vi "newMicroTime.vi"() -> ()   [LabVIEW 2013]
uses:
  Camera/vi/GlobalSetGetConfigureCamera.vi
  Variables/GetPicture.vi
  Variables/GlobalLaserInterface.vi
  Variables/patternImg.vi
panel:
  in  "Tab Control":T1(tab)
  out "Histogram":i32[][](graph)
  out "Trace":i32[][](graph)=[[2, 0, 0, 1, 1, 1, 0, 0, 0, 1, 0, 1, 0, 1, 2, 2, 0, 3, 0, 2, 2, 1, 3, 1, 0, 1, 1, 1, 0, 1, 3, 1, 0, 2, 0, 1, 0, 1, 1, 0, 1, 1, 3, 1, 0, 2, 0, 1, 1, 0, 0, 2, 0, 0, 1, 1, 1, 0, 0, 1, 0, 1, 0, 0, 0, 1, 2, 1, 1, 2, 0, 2, 4, 3, 1, 1, 0, 0, 1, 1, 2, 0, 1, 1, 0, 0, 0, 1, 1, 1, 1, 3, 0, 0, 1, 0, 0, 0, 2, 1, 1, 1, 2, 1, 0, 1, 1, 0, 0, 2, 1, 1, 0, 0, 1, 1, 1, 1, 0, 2, 2, 0, 1, 2, 1, 0, 3, 0, 2, 1, 3, 0, 1, 1, 0, 0, 3, 0, 0, 0, 0, 0, 0, 0, 0, 0, 0, 0, 0, 0, 0, 0, 0, 0, 0, 0, 0, 0, 0, 0, 0, 0, 0, 0, 0, 0, 0, 0, 0, 0, 0, 0, 0, 0, 0, 0, 0, 0, 0, 0, 0, 0, 0, 0, 0, 0, 0, 0, 0, 0, 0, 0, 0, 0, 0, 0, 0, 0, 0, 0], [1, 2, 2, 0, 0, 0, 1, 2, 1, 2, 1, 1, 1, 0, 0, 0, 3, 1, 0, 1, 0, 2, 0, 2, 1, 1, 0, 0, 1, 0, 1, 2, 1, 0, 0, 0, 0, 0, 1, 0, 1, 0, 2, 0, 1, 0, 0, 0, 0, 1, 1, 3, 0, 0, 0, 2, 0, 0, 2, 0, 1, 1, 0, 0, 2, 0, 2, 1, 0, 1, 1, 0, 1, 1, 0, 0, 0, 1, 0, 0, 1, 0, 0, 0, 0, 1, 0, 1, 1, 1, 1, 0, 0, 0, 1, 1, 1, 0, 1, 0, 0, 0, 1, 1, 1, 0, 0, 1, 1, 3, 1, 0, 0, 0, 0, 0, 0, 0, 1, 2, 1, 0, 0, 0, 2, 3, 3, 2, 0, 1, 1, 1, 0, 0, 4, 0, 1, 2, 0, 0, 0, 2, 0, 0, 0, 0, 0, 0, 0, 0, 0, 0, 0, 0, 0, 0, 0, 0, 0, 0, 0, 0, 0, 0, 0, 0, 0, 0, 0, 0, 0, 0, 0, 0, 0, 0, 0, 0, 0, 0, 0, 0, 0, 0, 0, 0, 0, 0, 0, 0, 0, 0, 0, 0, 0, 0, 0, 0, 0, 0], [2, 2, 0, 1, 2, 0, 1, 0, 2, 3, 1, 0, 1, 0, 1, 0, 0, 0, 0, 2, 1, 0, 0, 2, 2, 0, 0, 0, 3, 0, 0, 2, 2, 2, 0, 3, 0, 3, 1, 3, 1, 3, 1, 0, 3, 1, 3, 3, 1, 1, 1, 1, 2, 0, 1, 0, 1, 1, 1, 3, 0, 2, 3, 1, 1, 1, 0, 1, 0, 1, 2, 3, 1, 2, 1, 3, 0, 2, 0, 2, 0, 1, 0, 2, 2, 1, 1, 3, 1, 2, 1, 1, 1, 3, 0, 0, 0, 0, 1, 1, 1, 0, 1, 0, 2, 1, 1, 0, 1, 0, 1, 2, 2, 2, 2, 0, 1, 0, 0, 0, 1, 1, 2, 0, 0, 1, 5, 2, 2, 0, 2, 0, 2, 2, 2, 0, 1, 0, 6, 0, 0, 0, 0, 0, 0, 0, 0, 0, 0, 0, 0, 0, 0, 0, 0, 0, 0, 0, 0, 0, 0, 0, 0, 0, 0, 0, 0, 0, 0, 0, 0, 0, 0, 0, 0, 0, 0, 0, 0, 0, 0, 0, 0, 0, 0, 0, 0, 0, 0, 0, 0, 0, 0, 0, 0, 0, 0, 0, 0, 0], [0, 0, 1, 0, 1, 1, 0, 0, 0, 1, 1, 0, 1, 0, 0, 0, 0, 0, 2, 0, 0, 0, 0, 2, 0, 0, 0, 1, 1, 2, 1, 1, 1, 2, 1, 0, 0, 3, 0, 1, 1, 0, 0, 0, 0, 1, 0, 0, 2, 1, 0, 0, 1, 1, 1, 2, 2, 0, 1, 0, 0, 1, 0, 1, 1, 0, 0, 2, 1, 1, 2, 1, 1, 0, 0, 0, 0, 2, 1, 0, 0, 0, 0, 1, 0, 1, 0, 0, 0, 0, 1, 0, 0, 0, 0, 1, 0, 1, 1, 1, 0, 2, 3, 1, 1, 0, 1, 1, 1, 0, 1, 0, 0, 1, 1, 0, 2, 0, 0, 0, 0, 3, 0, 0, 0, 0, 0, 0, 0, 0, 1, 0, 2, 0, 0, 0, 1, 2, 2, 0, 1, 0, 0, 0, 0, 0, 0, 0, 0, 0, 0, 0, 0, 0, 0, 0, 0, 0, 0, 0, 0, 0, 0, 0, 0, 0, 0, 0, 0, 0, 0, 0, 0, 0, 0, 0, 0, 0, 0, 0, 0, 0, 0, 0, 0, 0, 0, 0, 0, 0, 0, 0, 0, 0, 0, 0, 0, 0, 0, 0]]
  out "Image":i32[][](graph)
  out "Video":u8[][](graph)
  out "AM image":T2(plugin-control)
  out "Auto Meas Progress":i32(slide) caption="Point 1 / 1" scale=0.0..1.0
  in  "Auto Meas":bool
  in  "Auto Measurement Time (ms)":i32=60 caption="Measurement Time (s)" min=10
  in  "Auto Shutter Control":bool=TRUE
  in  "Autopoint-Autofocus Z":bool=TRUE
  in  "Save Color Image":bool
  in  "Find Mols":bool
  in  "psf width [um]":dbl=0.7
  out "Pixel Y":dbl
  out "Pixel X":dbl
  in  "Aquire Image":bool
  out "Measure. time":dbl format="%7.1f s"
  in  "Picture size Y":dbl=50.0 min=0.1 max=200.0 format="%1.1f um"
  in  "Picture size X":dbl=50.0 min=0.1 max=200.0 format="%1.1f um"
  in  "Pixel time":dbl=1.0 min=0.1 max=10.0 step=0.1 format="%.1f ms"
  in  "Resolution":dbl=1.0 min=0.05 max=10.0 step=0.05 format="%.2f µm"
  in  "Axis":enum32{"x-y", "x-z", "y-x", "y-z", "z-x", "z-y"}(ring)
  in  "Grid Measurement":bool
  in  "Z-Axis Offset":dbl=2.0 min=0.1 max=10.0
  in  "Y-Axis Offset":dbl=2.0 min=0.1 max=10.0
  in  "X-Axis Offset":dbl=2.0 min=0.1 max=10.0
  in  "Z-Axis Points":u16=1 min=1 max=100
  in  "Y-Axis Points":u16=50 min=1 max=100
  in  "X-Axis Points":u16=50 min=1 max=100
  in  "Line Scan":bool
  in  "Measurement Time":i32=60 min=10 format="%.0d s"
  in  "Adjustment":bool
  in  "Move into solution":bool=TRUE
  in  "Point Measurement":bool
  in  "SCANNER EMERGENCY":bool
  in  "Stop Program":bool
  out "Task":T3(ring)
  in  "Get Position":bool
  in  "Move Stage":bool
  in  "X-Position":dbl=48.0021 caption="X" min=0.0 max=200.0 step=0.1 format="%1.3f um"
  in  "Y-Position":dbl=19.9997 caption="Y" min=0.0 max=200.0 step=0.1 format="%1.3f um"
  in  "Z-Position":dbl=69.999 caption="Z" min=0.0 max=200.0 step=0.1 format="%1.3f um"
  out "x-position":dbl format="%.3f"
  out "y-position":dbl format="%.3f"
  out "z-position":dbl format="%.3f"
  in  "CFD Settings":T4={"Sync Level"=15, "Sync ZeroX"=0, "Sync Offset"=0, "Chan Settings"=[{"CHx Level"=50, "CHx ZeroX"=10, "CHx Offset"=-22150}, {"CHx Level"=50, "CHx ZeroX"=10, "CHx Offset"=-21850}, {"CHx Level"=75, "CHx ZeroX"=10, "CHx Offset"=-6000}, {"CHx Level"=75, "CHx ZeroX"=10, "CHx Offset"=-5700}], "Laser  Profile"="1"}
  in  "Save Files":bool=TRUE
  in  "New MSW":bool
  in  "Open MSW":bool
  out "Workspace":path=path "X:/MTusers/Christoph/2011-02-01 Andi/2011-02-01.msw"
  in  "WS File Tree":string(tree)
  in  "Sample description":string
  out "error out":errorcluster
  out "Excitation":bool
  out "Detector 1":bool
  out "Detector 2":bool
  out "Intensity (a.u.)":string
  out "Auto Measure Points":i32
  out "NxtAutMesPoint":i32
  out "Pattern":dbl[][](array[numeric])
  out "concatenated string":string
  out "Global Stop":bool=TRUE
  out "Stop Measurement":bool
  in  "PI SystemNumber":i32=1
  in  "Image Measurent Parameters":T5
  out "Active pt3":path
  out "Buffer Overrun":bool
  out "Running":bool
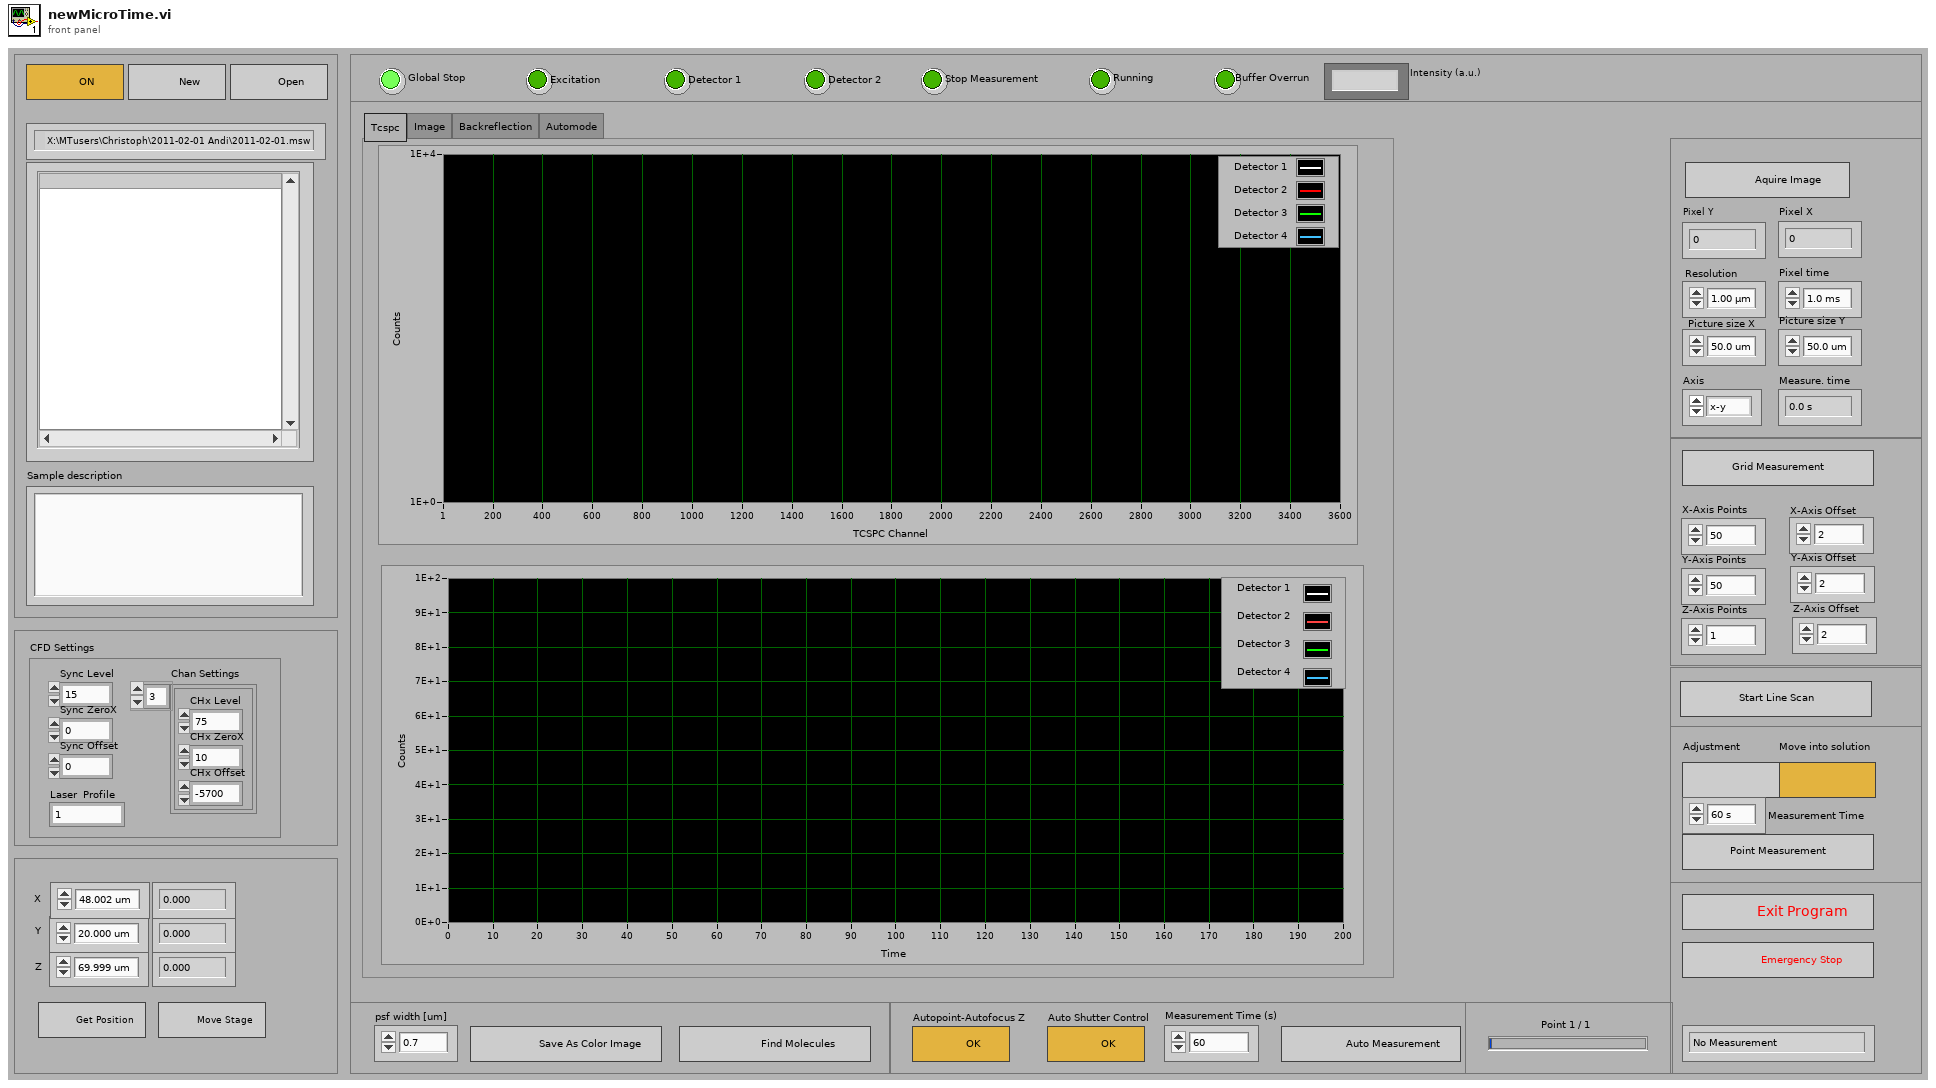
[diagram p1: front panel]
types:
  T1 = enum32{"Tcspc", "Image", "Backreflection", "Automode"}
  T2 = typedef "IMAQ Image.ctl" = refnum<image>
  T3 = enum16{"No Measurement", "Aquire Image", "Point Measurement", "Multi Measurement", "Save Color Image", "Find Single Mol.", "Auto Measurement Control", "Auto Point", "Aquire Line Scan", "Grid Measurement", "Trapping", "Move Scanner"}
  T4 = cluster{"Sync Level":i32, "Sync ZeroX":i32, "Sync Offset":i32, "Chan Settings":cluster{"CHx Level":i32, "CHx ZeroX":i32, "CHx Offset":i32}[], "Laser  Profile":string}
  T5 = cluster{"Position":cluster{"X-Position":dbl, "Y-Position":dbl, "Z-Position":dbl}, "Axis 1 Pixels":dbl, "Axis 2 Pixels":dbl, "Axis":i32, "Resolution":dbl, "PixelTime":dbl, "Laser pulses":i32}
  T6 = enum16{"CAN_Baud_1M", "CAN_BAUD_500K", "CAN_BAUD_250K", "CAN_BAUD_125K", "CAN_BAUD_100K", "CAN_BAUD_50K", "CAN_BAUD_20K", "CAN_BAUD_10K", "CAN_BAUD_5K", "User"}
  T7 = typedef "Image Type" = u32
  T8 = cluster{"Height":u32, "Width":u32, "Pixel Depth":u32}
  T9 = enum32{"TCSPC Histogram", "Trace", "Backreflection", "Image", "AutoMesaurement"}
  T10 = cluster{"ID":u32, "MSG type":enum8{"STD, NO RTR", "STD,RTR", "XTD, NO RTR", "XTD, RTR"}, "LEN":u8, "DATA":u8[]}
  T11 = cluster{"Dev":i32, "SerNo":string, "HW_Model":string, "HW_Partno":string}[]
  T12 = enum16{"No Measurement", "Aquire Image", "Point Measurement", "Multi Measurement", "Save Color Image", "Find Single Mol.", "Auto Measurement Control", "Auto Point", "Aquire Line Scan", "Grid Measurement"}
  T13 = enum16{"none", "fast axis", "slow axis", "both axis", ""}
  T14 = enum16{"none", "fast axis", "slow axis", "both", ""}
  T15 = enum16{"target position", "relative position", "actual position", "position error"}
  T16 = enum16{"not a pt3 File", "Image File", "Point Measurement", "Auto Point"}
  T17 = enum16{"unknown", "pt3 File", "png Image", "bmp Image"}
  T18 = enum16{"No Measurement", "Aquire Image", "Point Measurement", "Multi Measurement", "Save Color Image", "Find Single Mol.", "Auto Measurement Control", "Auto Point"}
  T19 = enum32{"TCSPC Histogram", "Trace", "Trapping", "CCD", "Backreflection", "Image", "AutoMesaurement"}
  T20 = enum16{"not a pt3 File", "Image File", "Point Measurement", "Auto Point", "Line Scan"}
  T21 = cluster{"Dev":i32, "SerNo":string, "HW_Model":string, "HW_Partno":string}
  T22 = cluster{"Comment":string, "Binning":i32, "Offset":i32, "AcquisitionTime (ms)":i32, "HardwareSerial":i32, "SyncDivider":i32, "Resolution (ps)":dbl, "CFD Settings":cluster{"Sync Level":i32, "Sync ZeroX":i32, "Sync Offset":i32, "Chan Settings":cluster{"CHx Level":i32, "CHx ZeroX":i32, "CHx Offset":i32}[]}, "ModuleInfo":cluster{"modelcode":i32, "versioncode":i32}[], "BaseResolution (ps)":dbl, "RefClockSource":i32, "ChanInfo":cluster{"CHx Level":i32, "CHx ZeroX":i32, "CHx Offset":i32, "CHx modidx":i32}[], "SyncRate":i32, "InputsEnabled":i64}
  T23 = cluster{"Dimensions":i32, "Time Per Pixel [ms]":dbl, "Acceleration":i32, "Pattern":i32, "X0":sgl, "Y0":sgl, "Z0":dbl, "PixX":i32, "PixY":i32, "PixResol":sgl, "TStartTo":sgl, "TStoptTo":sgl, "TStartFro":sgl, "TStopFro":sgl}
  T24 = cluster{"InpRateFilePos":i64, "StopAfterFilePos":i64}
  T25 = cluster{"X-Position":dbl, "Y-Position":dbl, "Z-Position":dbl}
  T26 = cluster{"File No":i32, "File Path":path, "Parent File":i32, "File Type":enum16{"unknown", "pt3 File", "png Image", "bmp Image"}, "Measurement Type":enum16{"not a pt3 File", "Image File", "Point Measurement", "Auto Point", "Line Scan", "Grid Scan"}, "Upper Left":cluster{"x-Position":dbl, "y-Position":dbl, "z-Position":dbl}, "Pixels":i32[], "Scan Axis":enum32{"x-y", "x-z", "y-z"}, "Resolution":dbl, "PixelTime":dbl}
  T27 = enum16{"not a pt3 File", "Image File", "Point Measurement", "Auto Point", "Line Scan", "Grid Scan"}
  T28 = cluster{"Ident":string, "Format Version":string, "Creator Name":string, "Creator Version":string, "File Time":string, "Comment":string, "Laser":i32, "Binning":i32, "Offset":i32, "AcquisitionTime (ms)":i32, "HardwareSerial":i32, "SyncDivider":i32, "Resolution (ps)":dbl, "Rates":dbl[], "SyncRate":dbl, "CFD Settings":cluster{"Sync Level":i32, "Sync ZeroX":i32, "Sync Offset":i32, "Chan Settings":cluster{"CHx Level":i32, "CHx ZeroX":i32, "CHx Offset":i32}[]}}
  T29 = cluster{"x-Position":dbl, "y-Position":dbl, "z-Position":dbl}
  T30 = enum16{"No Measurement", "Aquire Image", "Point Measurement", "Multi Measurement", "Save Color Image"}
  T31 = enum16{"No Measurement", "Aquire Image", "Point Measurement", "Multi Measurement", "Save Color Image", "Find Single Mol.", "Auto Measurement Control", "Auto Point", "Aquire Line Scan"}
  T32 = enum16{"No Measurement", "Aquire Image", "Point Measurement", "Multi Measurement", "Save Color Image", "Find Single Mol."}
  T33 = enum16{"Get (Default)", "Set Workspace", "Append File", "Change Comment"}
  T34 = cluster{"File No":i32, "File Path":path, "Parent File":i32, "File Type":enum16{"unknown", "pt3 File", "png Image", "bmp Image"}, "Measurement Type":enum16{"not a pt3 File", "Image File", "Point Measurement", "Auto Point", "Line Scan", "Grid Scan"}, "Upper Left":cluster{"x-Position":dbl, "y-Position":dbl, "z-Position":dbl}, "Pixels":dbl[], "Resolution":dbl, "Scan Axis":enum32{"x-y", "x-z", "y-x", "y-z", "z-x", "z-y"}, "PixelTime":dbl}[]
  T35 = cluster{"File No":i32, "File Path":path, "Parent File":i32, "File Type":enum16{"unknown", "pt3 File", "png Image", "bmp Image"}, "Measurement Type":enum16{"not a pt3 File", "Image File", "Point Measurement", "Auto Point", "Line Scan", "Grid Scan"}, "Upper Left":cluster{"x-Position":dbl, "y-Position":dbl, "z-Position":dbl}, "Pixels":i32[], "Scan Axis":enum32{"x-y", "x-z", "y-x", "y-z", "z-x", "z-y"}, "Resolution":dbl, "PixelTime":dbl}[]
  T36 = cluster{"File No":i32, "File Path":path, "Parent File":i32, "File Type":enum16{"unknown", "pt3 File", "png Image", "bmp Image"}, "Measurement Type":enum16{"not a pt3 File", "Image File", "Point Measurement", "Auto Point", "Line Scan", "Grid Scan"}, "Upper Left":cluster{"x-Position":dbl, "y-Position":dbl, "z-Position":dbl}, "Pixels":i32[], "Resolution":dbl, "Scan Axis":enum32{"x-y", "x-z", "y-z"}, "PixelTime":dbl}[]
  T37 = typedef "LVPoint32TypeDef.ctl" = cluster{"Horizontal":i32, "Vertical":i32}
  T38 = cluster{"Shift":bool, "Ctrl":bool, "Alt":bool, "Cmd":bool, "Opt":bool}
  T39 = cluster{"ID":u32, "MSG type":enum8{"STD, NO RTR", "STD,RTR", "XTD, NO RTR", "XTD, RTR"}, "LEN":u8, "Data":u8[]}
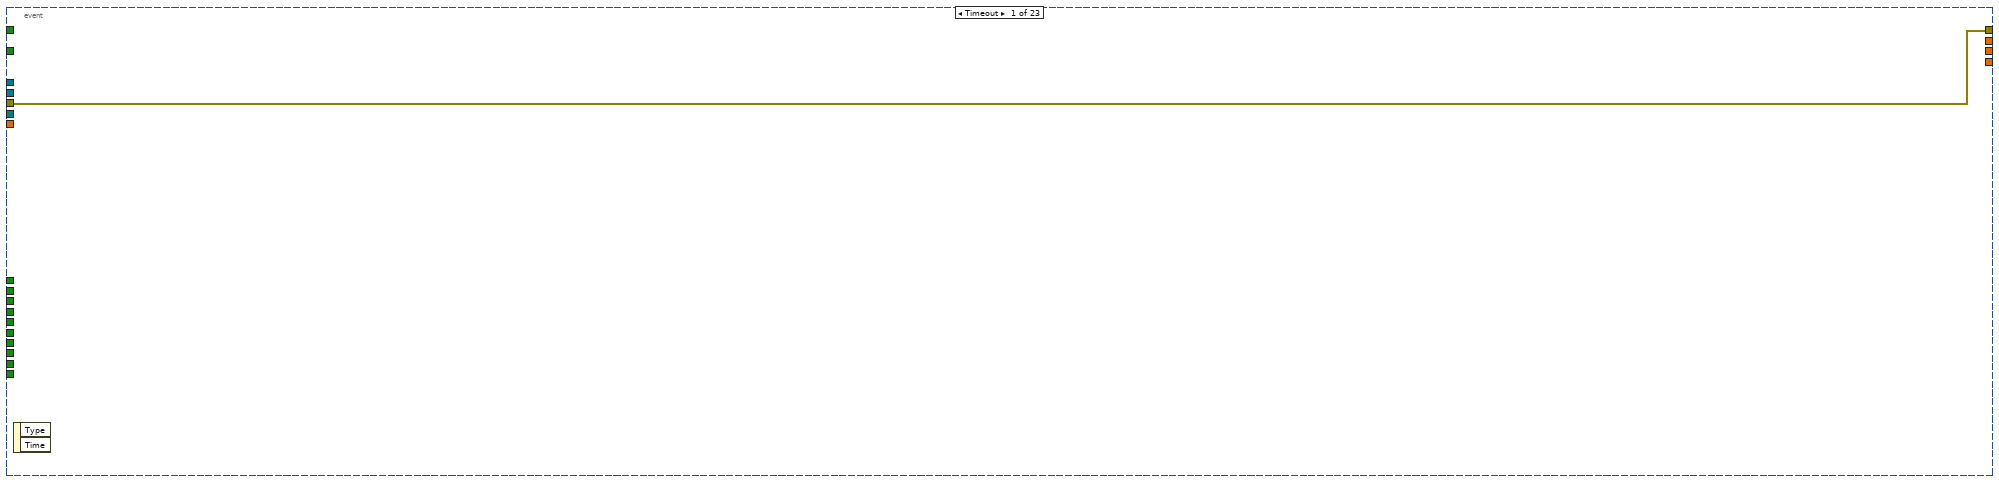
[diagram p3: hidden frame]
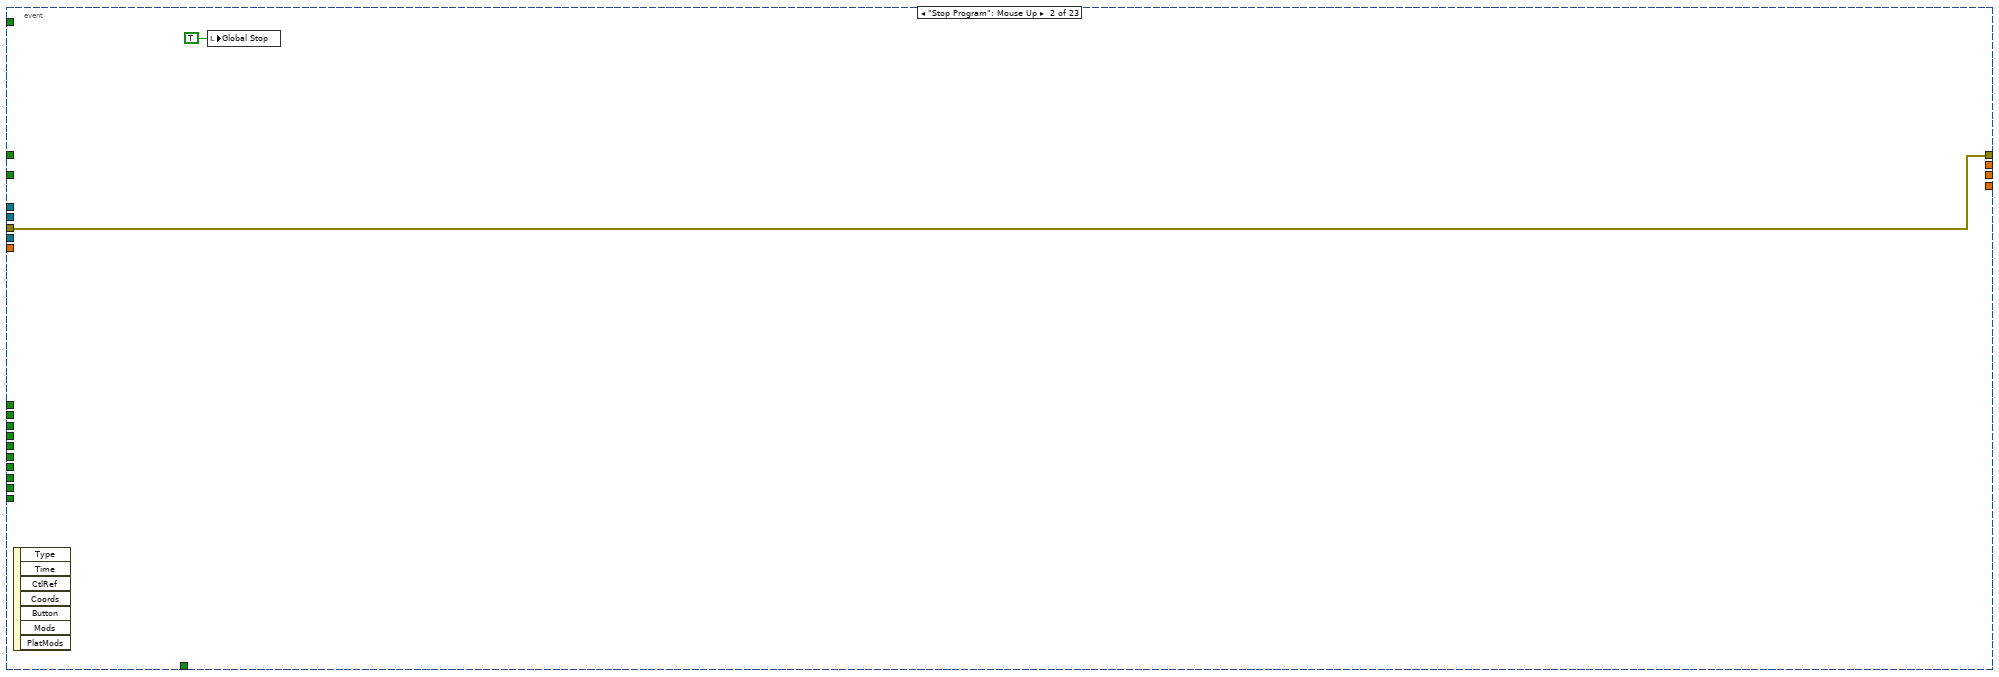
[diagram p4: hidden frame]
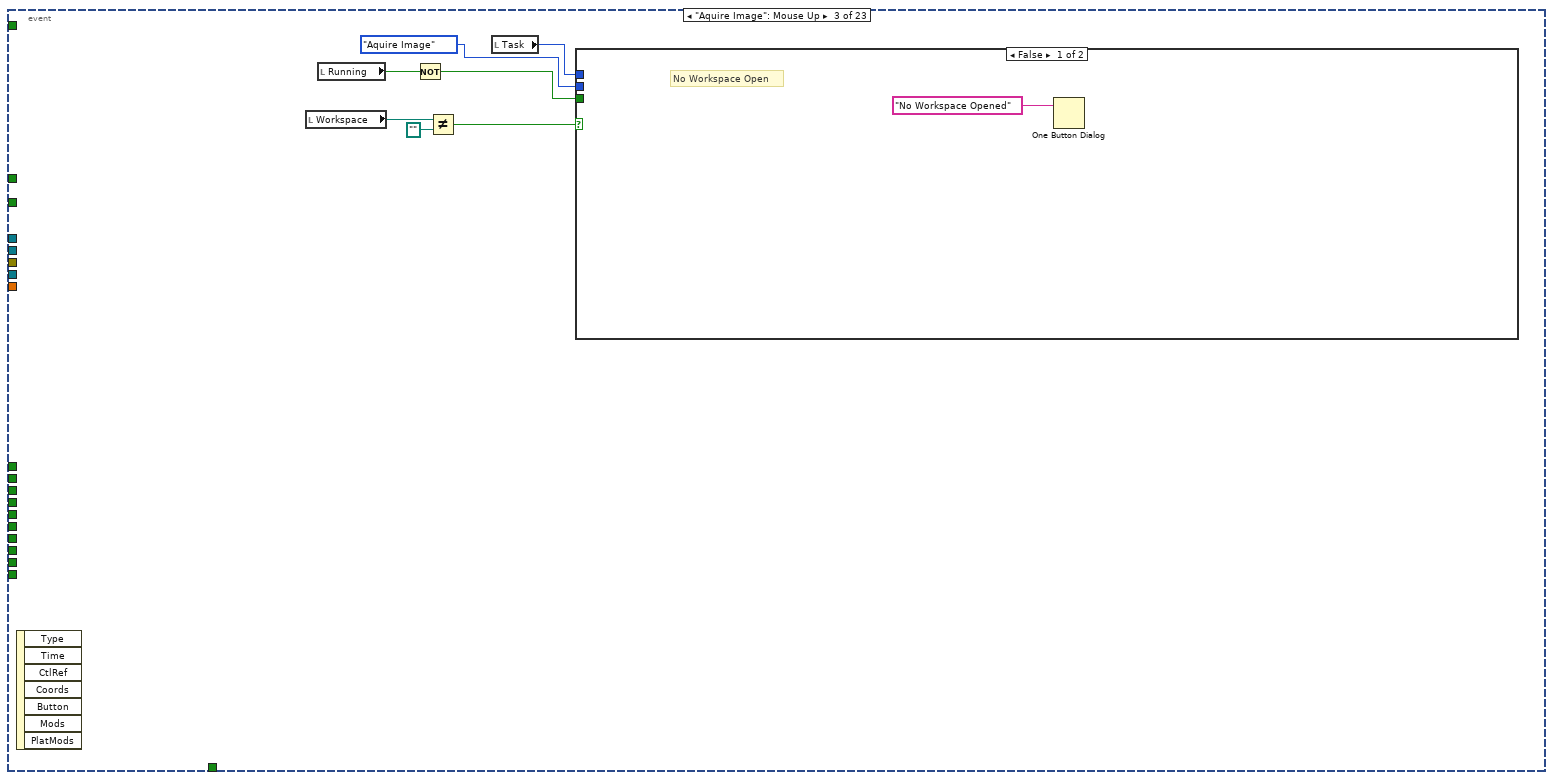
[diagram p5: hidden frame]
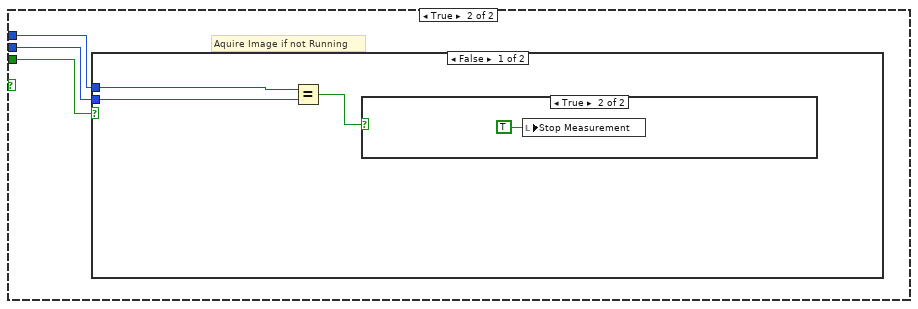
[diagram p6: hidden frame]
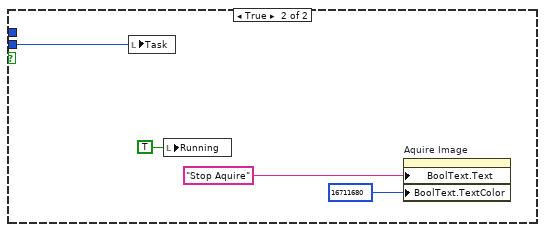
[diagram p8: hidden frame]
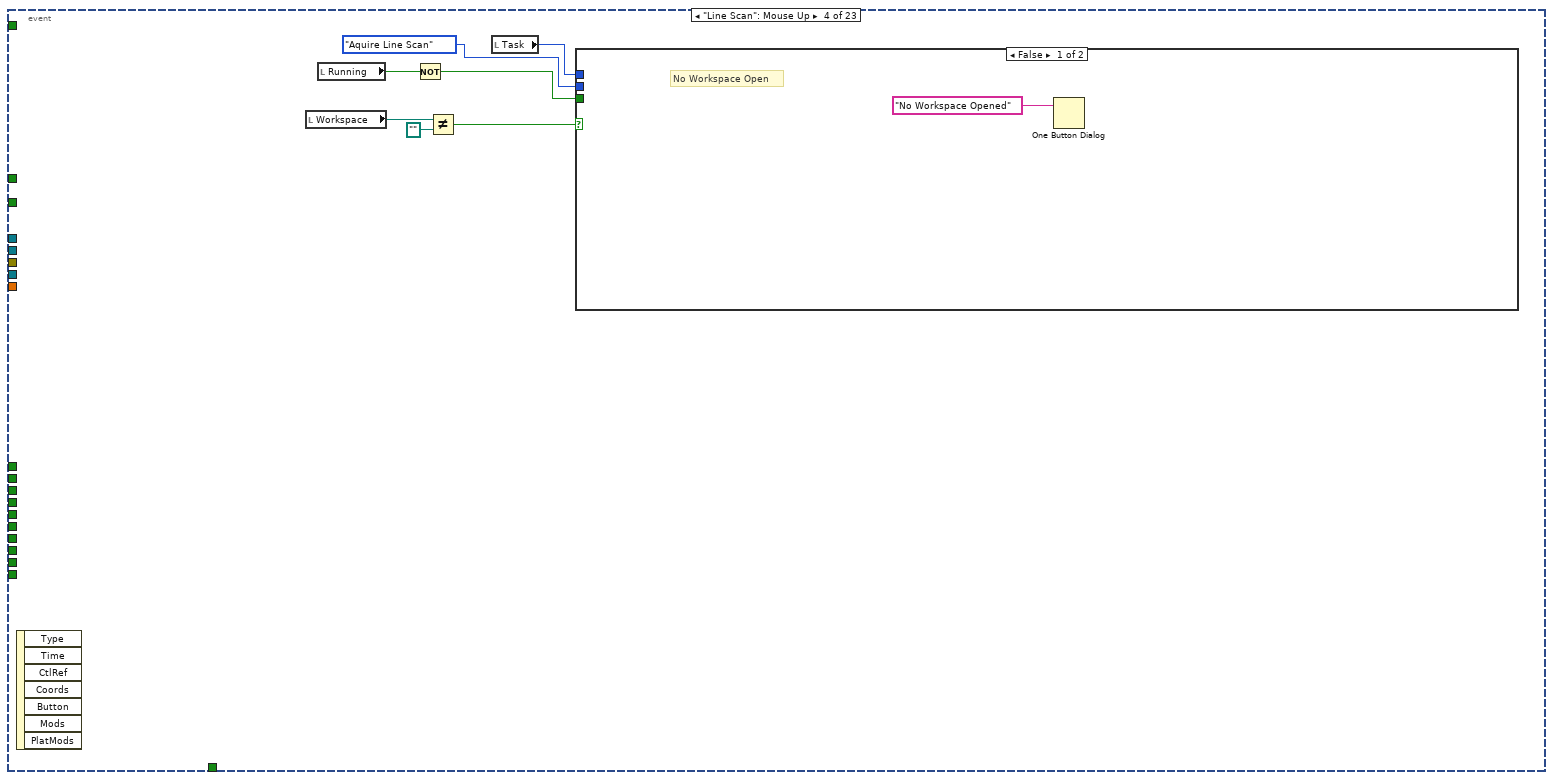
[diagram p9: hidden frame]
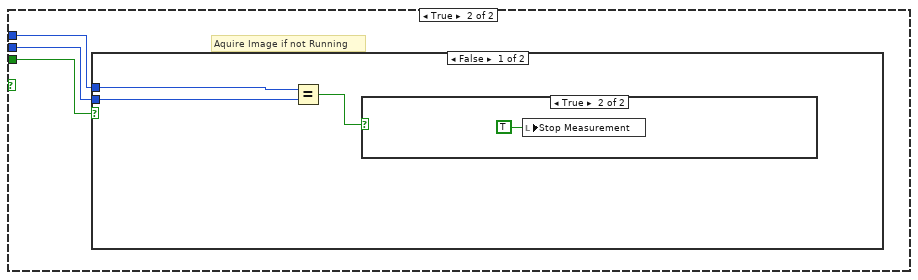
[diagram p10: hidden frame]
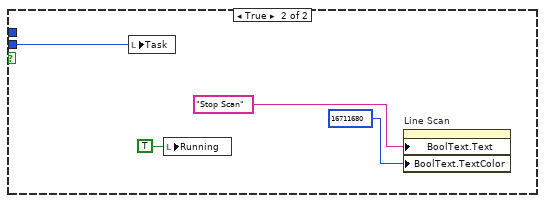
[diagram p12: hidden frame]
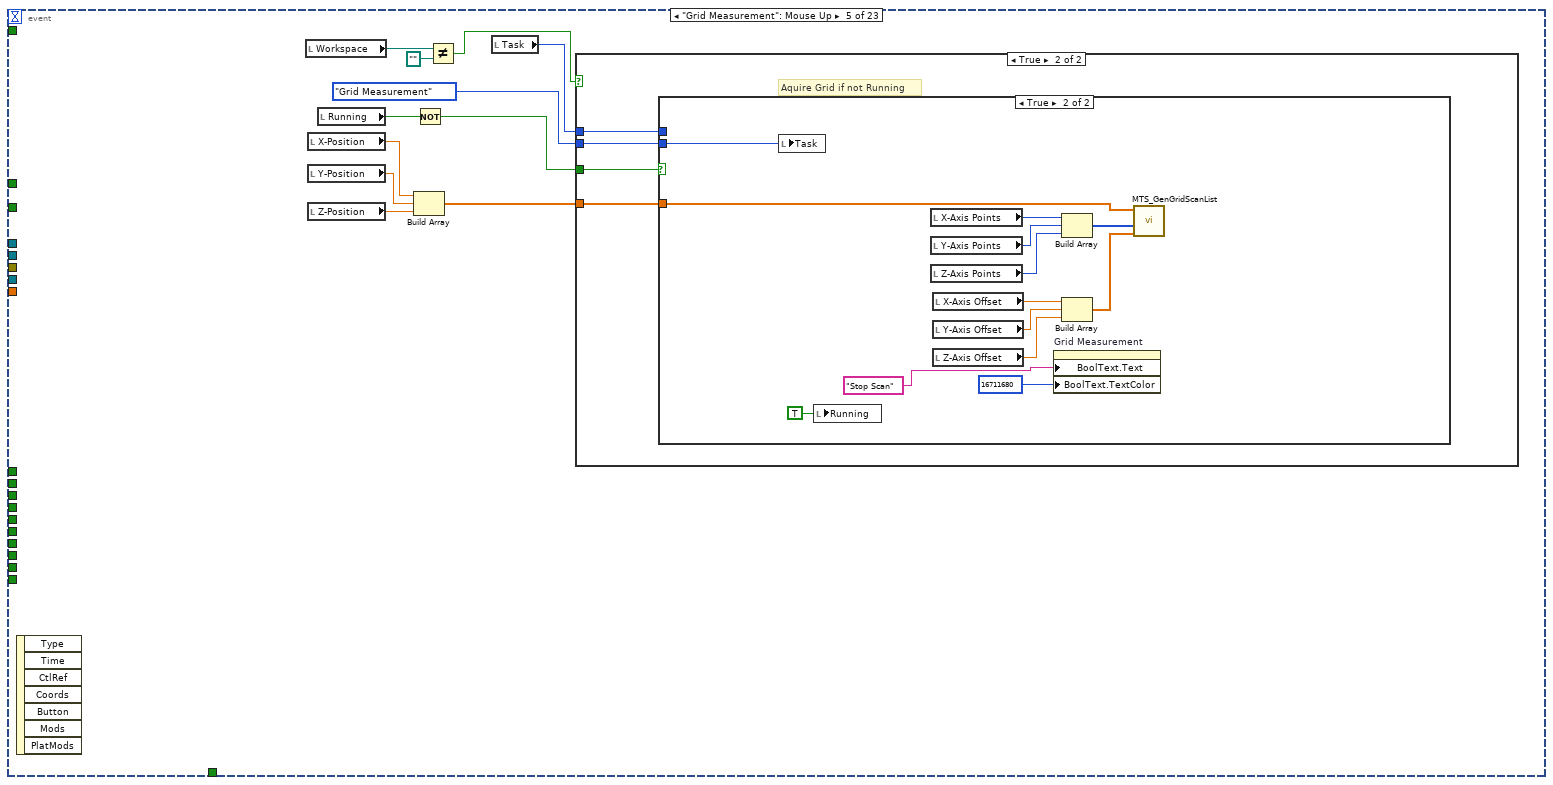
[diagram p13: hidden frame]
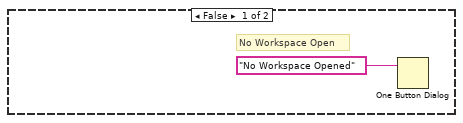
[diagram p14: hidden frame]
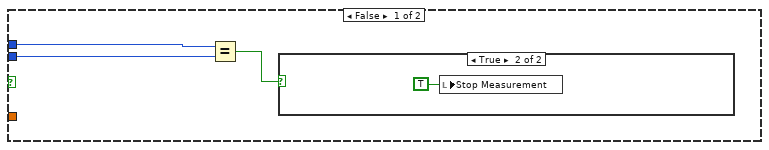
[diagram p15: hidden frame]
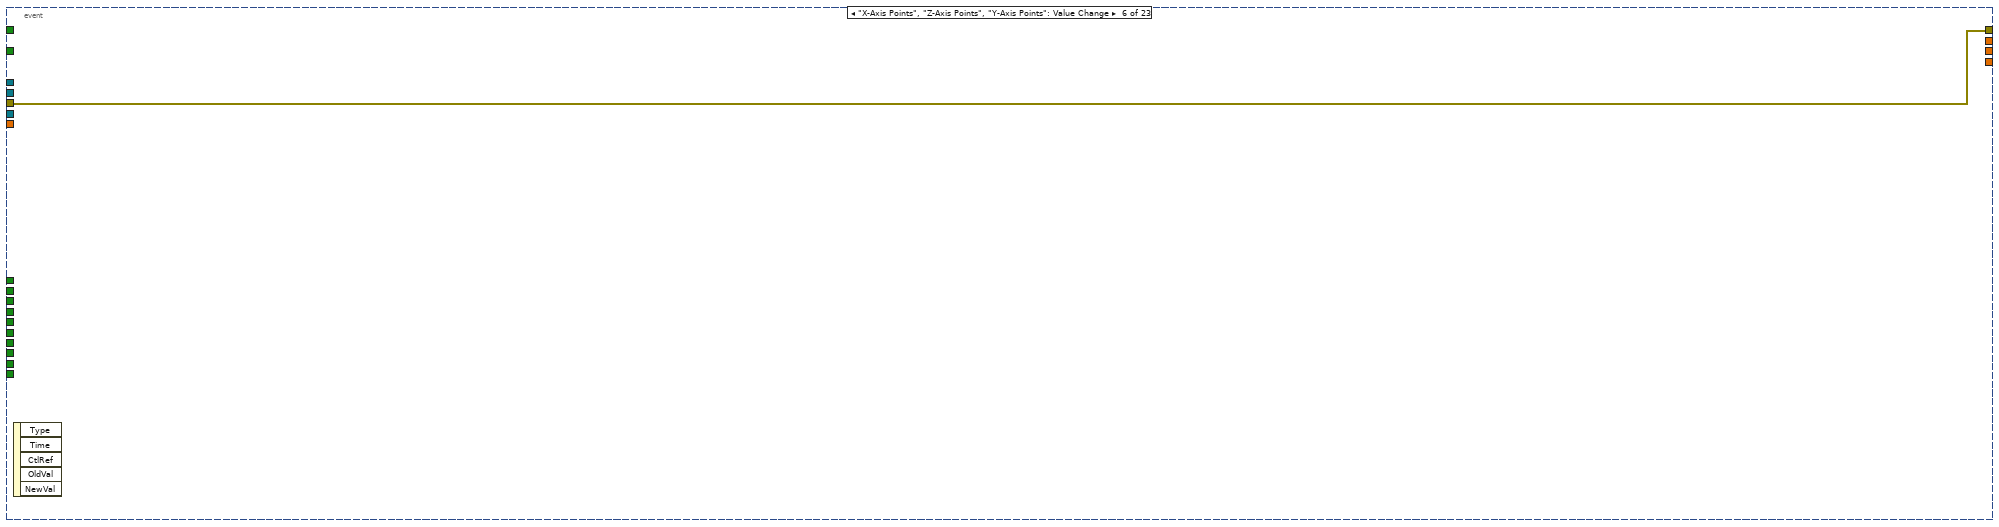
[diagram p17: hidden frame]
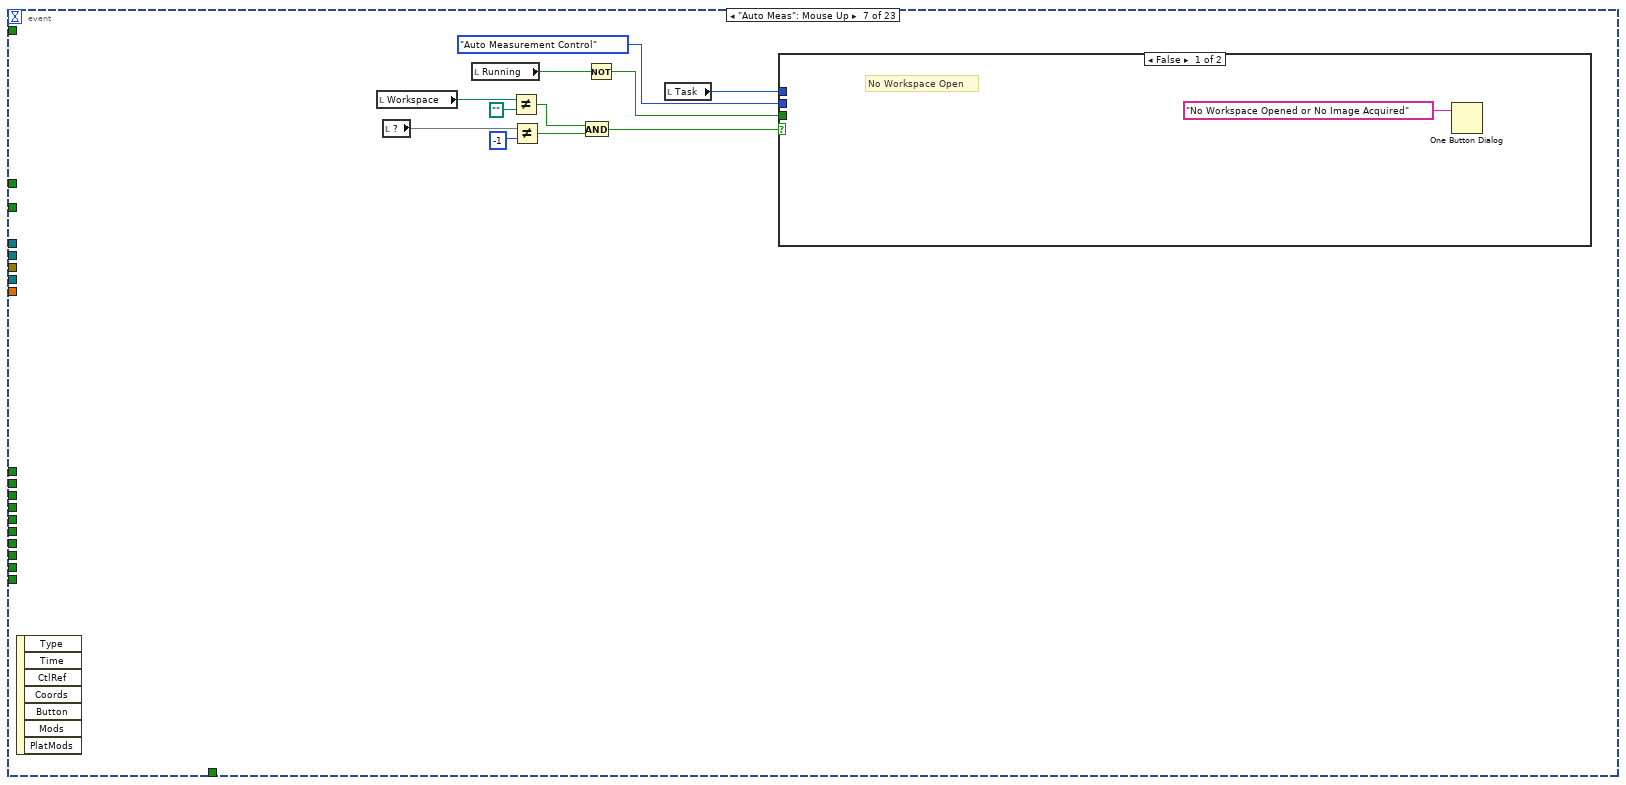
[diagram p18: hidden frame]
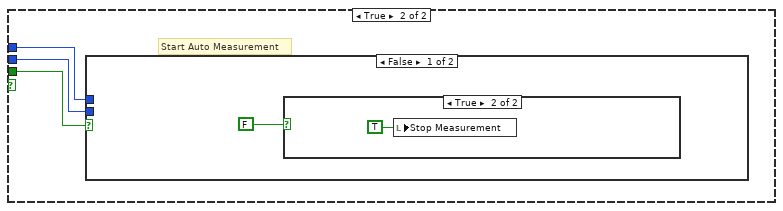
[diagram p19: hidden frame]
diagram:
  (unwired) "Please set the recording time to a positive value." ("message")
  (unwired) "Calibration forbidden when modulation is turned on." ("message")
  (unwired) "Modulation Frequency: %f Hz\nNumber of Modulation Points: %d\nModulation Radius: %f um\nModulation Angle: %f degrees\n" ("format string")
  (unwired) i8 4  # Variance Scale
  (unwired) "Scan Frequency: %f Hz\nBin Period: %f ns\nScan Form: %s\nPoints Per Scan: %d\nPoint Spacing: %f um\nSub-Bin Delay: %f ns\nBeam Waist: %f um\nEOD Scale: %f um/V\nDiffusion Constant: %f um^2/s\nMobility: %f um/s/V\nMaximum Feedback: %f V\nInclude Mobility Update: %s\n" ("format string")
  (unwired) "Must be in trapping mode for data storage." ("message")
  (unwired) "Please enter a new prefix." ("message")
  w23 = 41.0  # Shortest Bin Length (ticks)
  w24 = 40000000.0  # Clock Speed
  (unwired) u8 32  # Maximum Allowed Points
  # "Command Interpreter\nValue in 8 MSBs sets the command\n[Bracketed commands are deprecated]\n0, dflt - unrecognized\n1 - Go/Stop (T/F) (value in 16 LSBs)\n[2 - Acquire/stop acquiring (T/F) (value in 16 LSBs)]\n4 - Mobility Update? (value in 16 LSBs)\n5 - Inverse Diffusion Constant (value in 24 LSBs)\n6 - Inverse Mobility (value in 24 LSBs)\n7 - Saturated Position Step (value in 24 LSBs)\n8 - Bin Length in ticks (value in 24 LSBs)\n9 - Bins per Cycle (value in 8 LSBs)\n[10 - Bin Delay (T/F) (value in 16 LSBs)]\n11 - Sub-Bin Delay in ticks (value in 16 LSBs)\n12 - Cycles per Modulation (value in 24 LSBs)\n13 - Number of Modulation Points (value in 8 LSBs)\n16 - EOD Voltage (x) (value in 16 LSBs, address in bits 16-23)\n17 - EOD Voltage (y) (value in 16 LSBs, address in bits 16-23)\n[18 - Feedback Voltage (x) (value in 16 LSBs, address in bits 16-23)]\n[19 - Feedback Voltage (y) (value in 16 LSBs, address in bits 16-23)]\n20 - Modulation (x) (value in 16 LSBs, address in bits 16-23)\n21 - Modulation (y) (value in 16 LSBs, address in bits 16-23)"
  # "Maximum Voltage"
  # "Global Constants"
  n1 = flat-sequence {
    tunnel: [w53] -> w14
    tunnel: errorcluster {"status"=FALSE, "code"=0, "source"=""} ("error in") -> [w58]
    tunnel: [w31] -> w13
    tunnel: [w30] -> w12
    frame #0 {
      w35 = T7 0 items=["Grayscale (U8)", "Grayscale (I16)", "Grayscale (SGL)", "Complex (CSG)", "RGB (U32)", "HSL (U32)", "RGB (U64)", "Grayscale (U16)"] ("Image Type")
      w50 = T7 4 items=["Grayscale (U8)", "Grayscale (I16)", "Grayscale (SGL)", "Complex (CSG)", "RGB (U32)", "HSL (U32)", "RGB (U64)", "Grayscale (U16)"] ("Image Type")
      (unwired) 1.0 ("CCD Chip Vertical Start")
      w63 = path ""
      w70 = FALSE ("Global Stop")
      n2 = global write "GetPicture.vi" "GetPicture"(FALSE ("GetPicture")) -> ()
      n3 = local write item#-1(-1 ("Last Image File No")) -> ()
      n4 = control-ref of="WS File Tree"() -> (w69:refnum<vi>)
      n5 = property on="Line Scan" class="Bool"("BoolText.Text"="Start Line Scan" ("Caption.Text"), "BoolText.TextColor"=u32 0 ("Boolean Text.Colors:FG Color")) -> ()  [unwired: 2 in, 2 out]
      n6 = local write "PI SystemNumber"("PI SystemNumber") -> ()
      n7 = property on="Aquire Image" class="Bool"("BoolText.Text"="Aquire Image" ("Caption.Text"), "BoolText.TextColor"=u32 0 ("Boolean Text.Colors:FG Color")) -> ()  [unwired: 2 in, 2 out]
      n8 = call "CAN USB Init.vi"("CAN Msg Type"=enum16{"11 Bit (0)", "29/11 Bit (1)"}."29/11 Bit (1)", "BTR0BTR1"=T6."CAN_BAUD_500K") -> ("Error Number"=w39:u32)  [unwired: 7 in, 2 out]
      n9 = call "MTS_ClearWSTree2.vi"("error in"=w58, "Tree Refnum"=w69) -> ("error out"=w36:errorcluster)  [unwired: 8 in, 1 out]
      n10 = property on="Point Measurement" class="Bool"("BoolText.Text"="Point Measurement" ("Caption.Text"), "BoolText.TextColor"=u32 0 ("Boolean Text.Colors:FG Color")) -> ()  [unwired: 2 in, 2 out]
      n11 = call <vilib>:"Error Cluster From Error Code.vi"("error in (no error)"=w36, "error message (\"\")"="PCAN Init Error" ("error message (\"\")"), "error code (0)"=w39) -> ("error out"=w38:errorcluster)  [unwired: 6 in]
      n12 = property on="Grid Measurement" class="Bool"("BoolText.Text"="Grid Measurement" ("Caption.Text"), "BoolText.TextColor"=u32 0 ("Boolean Text.Colors:FG Color")) -> ()  [unwired: 2 in, 2 out]
      n13 = call "DT3120_InitDeviceList.vi"("error in (no error)"=w38) -> ("error out"=w48:errorcluster, "Alias List"=w49:string[])  [unwired: 9 out]
      n14 = Index Array(array=w49) -> (element=w47:string)  [unwired: 1 in]
      n15 = call "DT3120_NewDevice.vi"("error in (no error)"=w48, "Alias"=w47) -> ("error out"=w43:errorcluster, "DevId"=w42:i32)  [unwired: 8 out]
      n16 = call "DT3120_GetInputSourceList.vi"("error in (no error)"=w43, "DevId"=w42) -> ("error out"=w46:errorcluster, "Active Source"=w45:u16, "DevId (dup)"=w44:i32)  [unwired: 7 out]
      n17 = call "DT3120_GetFrameSize.vi"("error in (no error)"=w46, "Source"=w45, "DevId"=w44) -> ("error out"=w33:errorcluster, "Frame Size"=w30:T8, "DevId (dup)"=w31:i32)  [unwired: 6 in]
      n18 = call "IMAQ Create"("Image Name"="Video", "Image Type"=w35, "error in (no error)"=w33) -> ("error out"=w32:errorcluster)  [unwired: 2 in, 1 out]
      n19 = call "IMAQ Create"("Image Name"="Patternimg", "Image Type"=w50, "error in (no error)"=w32) -> ("New Image"=w51:T2, "error out"=w53:errorcluster)  [unwired: 2 in]
      n20 = global write "patternImg.vi" "New Image"(w51) -> ()
      n21 = global write "GlobalSetGetConfigureCamera.vi" "gain"(30 ("gain")) -> ()
      "Global Stop" <- w70
      "Running" <- w70
      "Buffer Overrun" <- w70
      "Stop Measurement" <- w70
      "Workspace" <- w63
      "Active pt3" <- w63
      "Task" <- T3."No Measurement" ("Do Measurement")
    }
  }
  n22 = control-ref of="X-Position"() -> (w19:refnum<vi>)
  n23 = control-ref of="Y-Position"() -> (w18:refnum<vi>)
  n24 = control-ref of="Z-Position"() -> (w17:refnum<vi>)
  n25 = local read "PI SystemNumber"() -> (w25:i32)
  n26 = control-ref of="PI SystemNumber"() -> (w20:refnum<vi>)
  n27 = while {
    shift-right: [w73] -> w9
    shift-left: w14 -> [w87]
    shift-right: [w80] -> _
    shift-left: w13 -> [w81]
    tunnel: w12 -> [w82]
    shift-right: [w79] -> w8
    shift-left: _ -> [w83]
    stop <- w86 stop-if-true
    n28 = local read "Running"() -> (w78:bool)
    n29 = Wait (ms)(milliseconds to wait=u32 100) -> ()  [unwired: 1 out]
    n30 = Equal?(x=T9."Backreflection" ("Tab Control")) -> (y=w72:T9, x = y?=w77:bool)
    n31 = Not(x=w78) -> (.not. x?=w75:bool)
    n32 = And(x=w77, y=w75) -> (x .and. y?=w76:bool)
    n33 = case shown="True" w76 {
      tunnel: w87 -> [w98 w106]
      tunnel: [w98 w105] -> w74
      tunnel: w83 -> [w96 w104]
      tunnel: w82 -> [_ w103]
      tunnel: w81 -> [w97 w102]
      tunnel: [w97 w101] -> w80
      tunnel: [w96 w100] -> w79
      frame False {
      }
      frame True {
        n34 = call "DT3120_AquireFrame.vi"("error in (no error)"=w106, "Image"=w104, "Frame Size"=w103, "DevId"=w102) -> ("error out"=w105:errorcluster, "Image Out"=w100:T2, "Frame"=→"Video":u8[][], "DevId (dup)"=w101:i32)  [unwired: 4 in]
      }
    }
    n35 = while {
      shift-right: [w90] -> w73
      shift-left: w74 -> [w90]
      stop <- w95 stop-if-true
      n36 = call "CAN USB Read.vi"() -> ("RcvQueueEmpty"=w95:bool, "CAN_Message out"=w94:T10)  [unwired: 1 in, 1 out]
      n37 = call "PCAN_DecompMessage.vi"("CAN_Message out"=w94) -> ("Intensity (a.u.)"=→"Intensity (a.u.)":dbl, "Detector2 Shutter Open?"=→"Detector 2":bool, "Detector1 Shutter Open?"=→"Detector 1":bool, "Excitation Shutter Open?"=→"Excitation":bool)  [unwired: 7 in]
    }
    n38 = local read "Global Stop"() -> (w85:bool)
    n39 = Unbundle(w73) -> ("status"=w84:bool)  [unwired: 2 out]
    n40 = Compound Arithmetic op=OR(w84, w85) -> (w86:bool)
  }
  n41 = call "AndorPhysikInstrumenteInitialisiation.vi"("reference"=w19, "error in (no error)"=w14, "reference 3"=w17, "reference 2"=w18, "Digital in"=w20) -> ("error out"=w16:errorcluster, "Device List"=w29:T11)  [unwired: 5 in]
  n42 = while {
    shift-right: [w114] -> w2
    shift-left: w16 -> [w111]
    tunnel: w25 -> [w122]
    tunnel: [w121] -> _
    shift-right: [w116] -> _
    shift-left: w16 -> [w123]
    tunnel: w29 -> [w115]
    tunnel: "Image Measurent Parameters" -> [w109]
    tunnel: [w108] -> _
    tunnel: "Sample description" -> [w107]
    stop <- w119 stop-if-true
    n43 = case shown="No Error" w111 {
      selector: w111 -> [w138 w810]
      tunnel: w123 -> [w150 w813]
      tunnel: w122 -> [w149 w814]
      tunnel: [w148 w814] -> w121
      tunnel: [w147 TRUE ("Global Stop")] -> w118
      tunnel: [w143 w813] -> w117
      tunnel: w115 -> [w142 _]
      tunnel: [w141 w810] -> w114
      tunnel: [w139 T12."No Measurement" ("Do Measurement")] -> w112
      tunnel: [w136 FALSE] -> w110
      tunnel: w109 -> [w135 _]
      tunnel: [w126 w810] -> w108
      tunnel: w107 -> [w124 _]
      frame No Error {
        n44 = while {
          shift-right: [w808] -> w144
          shift-left: w150 -> [w808]
          tunnel: [w803] -> w146
          tunnel: [w805] -> w145
          tunnel: [w804] -> w140
          stop <- w809 stop-if-true
          w804 = FALSE ("FiFo Overrun")
          # "Wait for Start"
          n45 = local read "Task"() -> (w803:T3)
          n46 = local read "Global Stop"() -> (w805:bool)
          n47 = Wait (ms)(milliseconds to wait=u32 100) -> ()  [unwired: 1 out]
          n48 = local write "Stop Measurement"(w804) -> ()
          n49 = Greater Than 0?(x=w803) -> (x > 0?=w807:bool)
          n50 = Or(x=w807, y=w805) -> (x .or. y?=w809:bool)
        }
        n51 = control-ref of="WS File Tree"() -> (w137:refnum<vi>)
        n52 = Build Array("X-Axis Points", "Y-Axis Points", "Z-Axis Points") -> (w131:u16[])
        n53 = Build Array("X-Axis Offset", "Y-Axis Offset", "Z-Axis Offset") -> (w127:dbl[])
        n54 = local write "Buffer Overrun"(w140) -> ()
        n55 = case shown="\"Auto Measurement Control\"" w146 {
          selector: w146 -> [_ _ w481 _ _ _]
          tunnel: w138 -> [w151 w191 w455 w638 w696 w757]
          tunnel: w149 -> [w156 w188 w418 w635 w695 w753]
          tunnel: [w156 w160 w418 w635 w695 w753] -> w148
          tunnel: [w151 w161 w422 w625 w693 w757] -> w141
          tunnel: [w152 FALSE ("Global Stop") FALSE ("Global Stop") FALSE ("Global Stop") FALSE ("Global Stop") FALSE ("Global Stop")] -> w147
          tunnel: w145 -> [w152 _ _ _ _ _]
          tunnel: w144 -> [w155 w174 w500 w637 w694 w758]
          tunnel: [w155 w174 w506 w637 w694 w756] -> w143
          tunnel: w142 -> [_ w246 w426 _ _ _]
          tunnel: [T12."No Measurement" ("Do Measurement") T12."No Measurement" ("Do Measurement") w480 T12."No Measurement" ("Do Measurement") T18."No Measurement" ("Do Measurement") w755] -> w139
          tunnel: w137 -> [_ _ w469 _ _ _]
          tunnel: [FALSE FALSE w461 FALSE _ _] -> w136
          tunnel: w135 -> [_ w223 _ _ _ _]
          tunnel: w131 -> [_ _ _ _ _ _]
          tunnel: w127 -> [_ _ _ _ _ _]
          tunnel: [w151 w194 w456 w625 _ _] -> w126
          tunnel: [_ _ w434 _ _ _] -> w125
          tunnel: w124 -> [_ _ w417 _ _ _]
          frame "No Measurement", Default {
          }
          frame "Aquire Image" {
            w184 = T20."Image File" ("Measurement Type")
            w227 = 32768 ("dimension size")
            # "TODO:\n- FIFO Read Flag Buffer Half Full?\n- auto square pixels"
            # "Image Intensity Array"
            n56 = Index Array(array=w246) -> (element=w245:T21)  [unwired: 1 in]
            n57 = Unbundle By Name(w245) -> ("Dev"=w214:i32)
            n58 = Index Array(array=string[] ["yx", "yz", "xy", "xz", "zy", "zx"] ("Array"), index="Axis") -> (element=w166:string)
            n59 = control-ref of="WS File Tree"() -> (w230:refnum<vi>)
            n60 = local read "Workspace"() -> (w235:path)
            n61 = control-ref of="Image"() -> (w208:refnum<vi>)
            n62 = String To Byte Array() -> (string=w164:string, unsigned byte array=w168:u8[])
            n63 = stacked-sequence {
              seq-local: [w258 _] -> [_ w285]
              seq-local: [w257 _] -> [_ w286]
              seq-local: [w256 _] -> [_ w281]
              seq-local: [w252 _] -> [_ w279]
              seq-local: [w253 _] -> [_ w278]
              seq-local: [w254 _] -> [_ w277]
              seq-local: [w250 _] -> [_ w273]
              tunnel: "Picture size X" -> [w271 _]
              tunnel: "Picture size Y" -> [w270 _]
              tunnel: w223 -> [w269 _]
              tunnel: "X-Position" -> [w268 _]
              tunnel: "Y-Position" -> [w267 _]
              tunnel: "Z-Position" -> [w266 _]
              tunnel: "Axis" -> [w260 _]
              tunnel: "Resolution" -> [w256 _]
              tunnel: [w259 _] -> w173
              tunnel: [_ w287] -> w192
              tunnel: w191 -> [w251 _]
              tunnel: w166 -> [_ w284]
              tunnel: w164 -> [_ w283]
              tunnel: "Pixel time" -> [w255 w282]
              tunnel: w188 -> [_ w280]
              tunnel: [_ w272] -> w187
              tunnel: [_ w276] -> w186
              tunnel: [_ w275] -> w185
              tunnel: [_ w274] -> w177
              frame #0 {
                n64 = call "PI_CheckScan.vi"("Picture size"=w271, "Picture size 2"=w270, "Axis"=w260, "x-Position"=w268, "y-Position"=w267, "z-Position"=w266, "error in (no error)"=w251) -> ("error out"=w250:errorcluster, "Picture size out"=w257:dbl, "Picture size out 2"=w258:dbl, "a0"=w252:dbl, "b0"=w253:dbl, "c0"=w254:dbl)  [unwired: 7 in]
                n65 = local write "Picture size X"(w257) -> ()
                n66 = local write "Picture size Y"(w258) -> ()
                n67 = Divide(x=w257, y=w256) -> (x/y=w263:dbl)
                n68 = Divide(x=w258, y=w256) -> (x/y=w264:dbl)
                n69 = Round Toward +Infinity(x=w263) -> (ceil(x): smallest int >= x=w262:dbl)
                n70 = Round Toward +Infinity(x=w264) -> (ceil(x): smallest int >= x=w261:dbl)
                n71 = Bundle("a0"=w252, "b0"=w253, "c0"=w254) -> (w265:cluster{"a0":dbl, "b0":dbl, "c0":dbl})  [unwired: 1 in]
                n72 = Bundle By Name(cluster=w269, "Position"=w265, "Axis 1 Pixels"=w262, "Axis 2 Pixels"=w261, "Axis"=w260, "Resolution"=w256, "PixelTime"=w255) -> (w259:T5)
              }
              frame #1 {
                n73 = call "PI_AreaScan_Prepare_1.vi"("System"=w280, "Laser"=w283, "Axis"=w284, "da"=w286, "db"=w285, "error in (no error)"=w273, "a0"=w279, "b0"=w278, "Resolution"=w281, "c0"=w277, "Pixel time"=w282) -> ("Tacq"=w272:dbl, "lp"=w275:i32, "ap"=w276:i32, "Trigger"=w274:dbl[], "error out"=w287:errorcluster)  [unwired: 4 in]
                "Measure. time" <- w272
              }
            }
            n74 = Unbundle By Name(w173) -> ("Axis 1 Pixels"=w201:dbl, "Axis 2 Pixels"=w202:dbl, "Resolution"=w199:dbl, "PixelTime"=w181:dbl)  [unwired: 2 out]
            n75 = Divide(x=w201, y=w199) -> (x/y=w210:dbl)
            n76 = Divide(x=w202, y=w199) -> (x/y=w212:dbl)
            n77 = call "HH_Set.vi"("Device List"=w246, "CFD Settings"="CFD Settings", "error in (no error)"=w192, "SyncDiv"=8) -> ("ht3 header out"=w206:T22, "Sync Rate"=w204:i32, "error out"=w176:errorcluster)  [unwired: 7 in, 2 out]
            n78 = Divide(x=w181, y=1000) -> (x/y=w179:dbl)
            n79 = Round Toward +Infinity(x=w210) -> (ceil(x): smallest int >= x=w209:dbl)
            n80 = Round Toward +Infinity(x=w212) -> (ceil(x): smallest int >= x=w211:dbl)
            n81 = call "MTS_PreapareImage.vi"("WS File Tree"=w230, "Workspace"=w235, "Measurement Type"=w184, "Image Measurent Parameters"=w173, "error in"=w176, "Trigger"=w177) -> ("File Name (dup)"=w219:path, "File No"=w228:i32, "Image Header"=w221:T23, "Comment"=w222:string, "error out"=w175:errorcluster)  [unwired: 5 in]
            n82 = Divide(x=1024, y=w204) -> (x/y=w183:dbl)
            n83 = local write "Active pt3"(w219) -> ()
            n84 = call "Scan_SetGraphScales.vi"("error in (no error)"=w175, "Image Measurent Parameters"=w173, "Image"=w208) -> ("error out"=w207:errorcluster)  [unwired: 8 in]
            n85 = Multiply(x=w187, y=1000) -> (x*y=w198:dbl)
            n86 = Subtract(x=w168, y=48) -> (x-y=w167:i32[])
            n87 = Initialize Array(0 ("element"), w209, w211) -> (w180:i32[][])
            n88 = Initialize Array(0, 5, 2) -> (w165:i32[][])
            n89 = Round Toward +Infinity(x=w198) -> (ceil(x): smallest int >= x=w196:dbl)
            n90 = Replace Array Subset(array=w165, new element=w167, index (col)=0) -> (w163:i32[][])  [unwired: 1 in]
            n91 = call "HT3_Create.vi"("Laser"=w163, "Image Header in"=w221, "Save pt3"="Save Files", "Measurement Type"=w184, "error in"=w207, "Comment"=w222, "ht3 Header in"=w206, "File Path"=w219) -> ("error out"=w236:errorcluster, "FileHeaderPos"=w226:T24, "refnum out"=w234:refnum<file>)  [unwired: 1 in]
            n92 = call "HH_Start.vi"("Device Index"=w214, "Acq. Time"=w196, "error in (no error)"=w236) -> ("error out"=w243:errorcluster)  [unwired: 11 in, 1 out]
            n93 = Unbundle By Name(w243) -> ("status"=w244:bool)
            n94 = Not(x=w244) -> (.not. x?=w242:bool)
            n95 = Initialize Array(u32 0, w227) -> (w239:u32[])
            n96 = case shown="True" w242 {
              tunnel: [w335 w366] -> w241
              tunnel: w188 -> [_ w361]
              tunnel: w243 -> [w336 w362]
              tunnel: w214 -> [w334 w353]
              tunnel: w180 -> [_ w338]
              tunnel: w239 -> [_ w360]
              tunnel: w227 -> [_ w359]
              tunnel: [w333 w358] -> w238
              tunnel: [w333 w357] -> w237
              tunnel: w234 -> [w332 w356]
              tunnel: [w332 w355] -> w233
              tunnel: [0 ("Num Records Total") w354] -> w232
              tunnel: [0.0 w347] -> w231
              tunnel: w166 -> [_ w350]
              tunnel: [dbl[] [] w344] -> w182
              tunnel: w179 -> [_ w340]
              tunnel: w177 -> [_ w339]
              frame False {
                (unwired) i32[][] [] ("Image Array Out")
                (unwired) u64[] [] ("Histograms")
                w333 = FALSE ("Stop Measurement")
                n97 = call "HH_Stop.vi"("Device Index"=w334, "error in (no error)"=w336) -> ("error out"=w335:errorcluster)  [unwired: 12 in, 1 out]
              }
              frame True {
                # "Overflow Interv. Time (s)"
                # "No Error"
                n98 = call "PI Start WG.vi"("System no."=w361, "axis"=w350, "Generator"=T13."both axis", "Init DDL"=T14."none", "increment"=T14."slow axis", "error in"=w362, "saved data"=T15."actual position") -> ("error out"=w363:errorcluster)  [unwired: 12 in]
                n99 = Initialize Array(0, 5) -> (w341:i32[])
                n100 = while {
                  tunnel: w353 -> [w386]
                  tunnel: w360 -> [w402]
                  tunnel: w359 -> [w401]
                  shift-right: [w387] -> w365
                  shift-left: w363 -> [w403]
                  shift-right: [FALSE ("Reset")] -> _
                  shift-left: TRUE ("Reset") -> [w374]
                  tunnel: [w395] -> w358
                  tunnel: [w391] -> w357
                  tunnel: w356 -> [w393]
                  tunnel: [w392] -> w355
                  tunnel: [w370] -> w354
                  tunnel: [w369] -> w347
                  shift-right: [w383] -> w346
                  shift-left: w341 -> [w381]
                  tunnel: [w380] -> w345
                  tunnel: w340 -> [w377]
                  tunnel: w339 -> [_]
                  shift-right: [w368] -> w337
                  shift-left: w338 -> [w376]
                  i -> [w379]
                  stop <- w400 stop-if-true
                  n101 = call "HH_FIFORead.vi"("Device Index"=w386, "Buffer In"=w402, "Count"=w401, "error in (no error)"=w403) -> ("OK"=w396:bool, "Buffer Out"=w373:u32[], "Data Count"=w372:i32, "FiFo Overrun"=w395:bool, "error out"=w394:errorcluster)  [unwired: 7 in]
                  n102 = local read "Stop Measurement"() -> (w390:bool)
                  n103 = local write "Buffer Overrun"(w395) -> ()
                  n104 = call "HT3_Write.vi"("error in"=w394, "Data Count"=w372, "Data in"=w373, "refnum in"=w393) -> ("error out"=w388:errorcluster, "refnum out"=w392:refnum<file>)  [unwired: 6 in]
                  n105 = Unbundle(w394) -> ("status"=w399:bool)  [unwired: 2 out]
                  n106 = local read "Global Stop"() -> (w389:bool)
                  n107 = call "GetCountRates.vi"("error in (no error)"=w388, "DeviceIndex"=w386) -> ("error out"=w387:errorcluster, "CntRates"=w385:dbl[], "SyncRate"=w378:i32)  [unwired: 1 in]
                  n108 = Multiply(x=w377, y=w378) -> (x*y=w367:dbl)
                  n109 = Compound Arithmetic op=OR(invert w396, w399, w389, w390) -> (w400:bool)
                  n110 = Insert Into Array(array=w385, index=0, new element=w378) -> (w382:dbl[])
                  n111 = call "HH_ToImage.vi"("Data In"=w373, "Reset"=w374, "Image Array In"=w376, "Data Count"=w372, "Pixel Time (Laser Pulses)"=w367) -> ("Image Array Out"=w368:i32[][], "Histograms"=→"Histogram":i32[][], "Total Oveflow Count"=w369:u64, "Num Records Total"=w370:i64, "Traces"=→"Trace":i32[][])  [unwired: 4 in, 2 out]
                  n112 = Or(x=w390, y=w389) -> (x .or. y?=w391:bool)
                  n113 = Add(x=w381, y=w382) -> (x+y=w383:dbl[])
                  n114 = Wait (ms)(milliseconds to wait=u32 2) -> ()  [unwired: 1 out]
                  n115 = Increment(x=w379) -> (x+1=w380:i32)
                }
                "Image" <- w337
                n116 = Divide(x=w346, y=w345) -> (x/y=w344:dbl[])
                n117 = call "HH_Stop.vi"("Device Index"=w353, "error in (no error)"=w365) -> ("error out"=w366:errorcluster)  [unwired: 12 in, 1 out]
              }
            }
            n118 = flat-sequence {
              tunnel: w241 -> [w306]
              tunnel: [w295] -> w193
              tunnel: w238 -> [w308]
              tunnel: w237 -> [w297]
              tunnel: w188 -> [w305]
              tunnel: [w304] -> w160
              tunnel: w233 -> [w302]
              tunnel: w232 -> [w301]
              tunnel: w231 -> [w291]
              tunnel: w226 -> [w296]
              tunnel: w183 -> [w292]
              tunnel: w182 -> [w288]
              frame #0 {
                # "Count Rate (per s)"
                # "Finish after Aquire Image"
                n119 = Multiply(x=w292, y=w291) -> (x*y=w290:dbl)
                n120 = Or(x=w297, y=w308) -> (x .or. y?=w307:bool)
                n121 = case shown="False" w307 {
                  tunnel: w306 -> [w313 w323]
                  tunnel: w305 -> [w311 w324]
                  tunnel: [w310 w324] -> w304
                  tunnel: [w312 w322] -> w303
                  tunnel: [enum16{"timeover", "manual", "overflow"}."timeover" ("Stop Reason") w327] -> w298
                  tunnel: w297 -> [w309 w325]
                  frame False {
                    # "Stop WaveGen\nif Aborted"
                    n122 = case shown="True" w309 {
                      tunnel: w313 -> [w315 w320]
                      tunnel: [w315 w319] -> w312
                      tunnel: w311 -> [w316 w318]
                      tunnel: [w316 w318] -> w310
                      frame False {
                      }
                      frame True {
                        n123 = call "PI Write GPIB.vi"("System no."=w318, "String to send"="0RT", "error in"=w320) -> ("error out"=w319:errorcluster)  [unwired: 16 in]
                      }
                    }
                  }
                  frame True {
                    n124 = Select(t=enum16{"timeover", "manual", "overflow"}."manual" ("Stop Reason"), s=w325, f=enum16{"timeover", "manual", "overflow"}."overflow" ("Stop Reason")) -> (s? t:f=w327:enum16{"timeover", "manual", "overflow"})
                    n125 = call "PI Write GPIB.vi"("System no."=w324, "String to send"="0RT", "error in"=w323) -> ("error out"=w322:errorcluster)  [unwired: 16 in]
                  }
                }
                n126 = Multiply(x=w290, y=1000.0) -> (x*y=w300:dbl)
                n127 = property on="Aquire Image" class="Bool"("BoolText.Text"="Aquire Image" ("Caption.Text"), "BoolText.TextColor"=u32 0 ("Boolean Text.Colors:FG Color")) -> ()  [unwired: 2 in, 2 out]
                n128 = To Long Integer(number=w300) -> (32bit integer=w299:i32)
                n129 = call "HT3_Finish.vi"("FileHeaderPos"=w296, "Rates"=w288, "Stop Reason"=w298, "error in"=w303, "Num Records"=w301, "Stop After (ms)"=w299, "refnum in"=w302) -> ("error out"=w295:errorcluster)  [unwired: 4 in]
              }
            }
            n130 = local read "X-Position"() -> (w157:dbl)
            n131 = local read "Y-Position"() -> (w158:dbl)
            n132 = local read "Z-Position"() -> (w159:dbl)
            n133 = call "AOTF-Trigger_1.vi"("Channel"=w164, "error in (no error)"=w192, "Triggered"=TRUE, "lp"=w185, "ap"=w186) -> ("error out"=w194:errorcluster)  [unwired: 2 in]
            n134 = call "PI Goto GPIB.vi"("System no."=w160, "x-position"=w157, "y-position"=w158, "z-position"=w159, "error in"=w193) -> ("error out"=w161:errorcluster)  [unwired: 14 in]
          }
          frame "Point Measurement", "Auto Point" {
            w429 = 0
            w467 = 32768 ("dimension size")
            n135 = Index Array(array=w426) -> (element=w511:T21)  [unwired: 1 in]
            n136 = property on="Measurement Time" class="DigNum (strict)" props=["Value"]() -> ()  [unwired: 2 in, 3 out]
            n137 = Unbundle By Name(w511) -> ("Dev"=w482:i32)
            n138 = case shown="False" "Move into solution" {
              tunnel: [0.0 40.0] -> w427
              frame False {
              }
              frame True {
              }
            }
            n139 = local read "Z-Position"() -> (w425:dbl)
            n140 = local read "Auto Shutter Control"() -> (w405:bool)
            n141 = local read "X-Position"() -> (w488:dbl)
            n142 = local read "Y-Position"() -> (w487:dbl)
            n143 = Add(x=w425, y=w427) -> (x+y=w424:dbl)
            n144 = Equal?(x=w481, y=T3."Auto Point" ("Task")) -> (x = y?=w462:bool)
            n145 = local read item#-1() -> (w473)
            n146 = And(x=w405, y=w462) -> ()  [unwired: 1 out]
            n147 = Select(t=T12."Auto Measurement Control" ("Do Measurement"), s=w462, f=T12."No Measurement" ("Do Measurement")) -> (s? t:f=w480:T12)
            n148 = And(x=w462, y="Autopoint-Autofocus Z") -> (x .and. y?=w468:bool)
            n149 = Bundle("X-Position"=w488, "Y-Position"=w487, w424) -> (w470:cluster{"X-Position":dbl, "Y-Position":dbl, dbl})  [unwired: 1 in]
            n150 = Select(t="AutoPoint" ("Measurement Type"), s=w462, f="Point" ("Measurement Type")) -> (s? t:f=w412:string)
            n151 = local read "concatenated string"() -> (w413:string)
            n152 = Select(t=T16."Auto Point" ("Measurement Type"), s=w462, f=T16."Point Measurement" ("Measurement Type")) -> (s? t:f=w475:T16)
            n153 = call "MTS_AutoPointCords.vi"("Is Auto Point"=w462, "Cords In"=w470) -> ("Cords"=w450:T25)  [unwired: 9 in]
            n154 = Select(t=w473, s=w462, f=-1) -> (s? t:f=w471:i32)
            n155 = Unbundle By Name(w450) -> ("X-Position"=w449:dbl, "Y-Position"=w447:dbl, "Z-Position"=w448:dbl)
            n156 = local read "Workspace"() -> (w498:path)
            n157 = Concatenate Strings(w413, w412) -> (w411:string)
            n158 = call "MTS_GenFileComment.vi"("Measurement Type"=w475, "Parent File No"=w471, "Info"=w417, "Upper Left"=w450, "error in"=w500) -> ("Comment"=w499:string, "error out"=w497:errorcluster)  [unwired: 7 in, 2 out]
            n159 = local read "PI SystemNumber"() -> (w410:i32)
            n160 = call "PI Goto GPIB.vi"("System no."=w418, "x-position"=w449, "y-position"=w447, "z-position"=w448, "error in"=w455) -> ("error out"=w409:errorcluster)  [unwired: 14 in]
            n161 = Select(t="Auto Measurement Time (ms)", s=w462, f="Measurement Time") -> (s? t:f=w465:i32)
            n162 = call "MTS_GetNextFileName.vi"("error in (no error)"=w497, "File Type"="ht3", "Measurement Type"=w411, "Workspace"=w498) -> ("error out"=w492:errorcluster, "Next File Name"=w491:path)  [unwired: 6 in]
            n163 = call "PI Pos GPIB.vi"("System no."=w410, "error in"=w409) -> ("error out"=w408:errorcluster)  [unwired: 14 in, 3 out]
            n164 = Not(x="Adjustment") -> (.not. x?=w415:bool)
            n165 = local read "CFD Settings"() -> (w460:T4)
            n166 = case shown="True" w415 {
              tunnel: w492 -> [w514 w522]
              tunnel: w491 -> [_ w521]
              tunnel: [w514 w520] -> w490
              tunnel: [path "D:/tmp.ht3" w515] -> w489
              tunnel: w475 -> [_ w517]
              tunnel: w471 -> [_ w519]
              tunnel: w469 -> [_ w516]
              frame False {
              }
              frame True {
                n167 = call "MTS_AddFileToWorkspace.vi"("File Name"=w521, "File Type"=T17."pt3 File", "Measurement Type"=w517, "error in (no error)"=w522, "Parent"=w519, "Tree Refnum"=w516) -> ("File Name (dup)"=w515:path, "error out"=w520:errorcluster)  [unwired: 7 in, 1 out]
              }
            }
            n168 = Multiply(x=w465, y=1000) -> (x*y=w464:i32)
            n169 = call "HH_Set.vi"("Device List"=w426, "CFD Settings"=w460, "error in (no error)"=w408) -> ("ht3 header out"=w486:T22, "Sync Rate"=w444:i32, "error out"=w484:errorcluster)  [unwired: 8 in, 2 out]
            n170 = Bundle By Name(cluster=w486, "AcquisitionTime (ms)"=w464) -> (w485:T22)
            n171 = Divide(x=65536 ("n"), y=w444) -> (x/y=w445:dbl)
            n172 = case shown="True" w468 {
              tunnel: w484 -> [w525 w532]
              tunnel: [w525 w531] -> w483
              tunnel: w482 -> [_ w530]
              tunnel: w445 -> [_ w529]
              tunnel: w450 -> [_ w528]
              frame False {
              }
              frame True {
                # "Auto Z"
                n173 = call "MTS_AutoZPos.vi"("PH Dev"=w530, "OFlow Interv [s]"=w529, "error in"=w532, "Start Point"=w528) -> ("New Z"=w527:dbl, "Counts"=w526:u32[], "error out"=w531:errorcluster)  [unwired: 9 in]
                n174 = local write "Z-Position"(w527) -> ()
              }
            }
            n175 = Initialize Array(u32 0, w467) -> (w504:u32[])
            n176 = flat-sequence {
              tunnel: w508 -> [w553]
              tunnel: w507 -> [w549]
              tunnel: [w553] -> w506
              tunnel: [w546] -> w423
              tunnel: w503 -> [w551]
              tunnel: w502 -> [w542]
              tunnel: w494 -> [w545]
              tunnel: w493 -> [w544]
              tunnel: w466 -> [w541]
              tunnel: w452 -> [w538]
              tunnel: w451 -> [w537]
              frame #0 {
                # "Finish after Measurement"
                n177 = Or(x=w542, y=w551) -> (x .or. y?=w550:bool)
                n178 = Index Array(array=w538, index=0) -> (element=w539:dbl)
                n179 = case shown="False" w550 {
                  tunnel: w549 -> [w555 w556]
                  tunnel: [w555 w556] -> w547
                  tunnel: [enum16{"timeover", "manual", "overflow"}."timeover" ("Stop Reason") w559] -> w543
                  tunnel: w542 -> [_ w557]
                  frame False {
                  }
                  frame True {
                    n180 = Select(t=enum16{"timeover", "manual", "overflow"}."manual" ("Stop Reason"), s=w557, f=enum16{"timeover", "manual", "overflow"}."overflow" ("Stop Reason")) -> (s? t:f=w559:enum16{"timeover", "manual", "overflow"})
                  }
                }
                n181 = Divide(x=w537, y=w539) -> (x/y=w536:dbl)
                n182 = Multiply(x=1024000, y=w536) -> (x*y=w534:dbl)
                n183 = To Long Integer(number=w534) -> (32bit integer=w533:i32)
                n184 = property on="Point Measurement" class="Bool"("BoolText.Text"="Point Measurement" ("Caption.Text"), "BoolText.TextColor"=u32 0 ("Boolean Text.Colors:FG Color")) -> ()  [unwired: 2 in, 2 out]
                n185 = call "HT3_Finish.vi"("FileHeaderPos"=w541, "Rates"=w538, "Stop Reason"=w543, "error in"=w547, "Num Records"=w544, "Stop After (ms)"=w533, "refnum in"=w545) -> ("error out"=w546:errorcluster)  [unwired: 4 in]
              }
            }
            n186 = local read item#-1() -> (w443)
            n187 = String To Byte Array(string=w443) -> (unsigned byte array=w441:u8[])
            n188 = Subtract(x=w441, y=48) -> (x-y=w436:i32[])
            n189 = String Length(string=w443) -> (length=w433:i32)
            n190 = Initialize Array(0, 5, 2) -> (w437:i32[][])
            n191 = Replace Array Subset(array=w437, new element=w436, index (col)=w429) -> (w435:i32[][])  [unwired: 1 in]
            n192 = Array Subset(array=w434, index=w429, length=w433) -> (w432:void[])
            n193 = local read "Auto Shutter Control"() -> (w404:bool)
            n194 = local read "X-Position"() -> (w421:dbl)
            n195 = local read "Y-Position"() -> (w419:dbl)
            n196 = local read "Z-Position"() -> (w420:dbl)
            n197 = Replace Array Subset(array=w435, new element=w432, index (col)=1) -> (w431:i32[][])  [unwired: 1 in]
            n198 = call "HT3_Create.vi"("Laser"=w431, "Save pt3"=w415, "error in"=w483, "Comment"=w499, "ht3 Header in"=w485, "File Path"=w489) -> ("error out"=w501:errorcluster, "FileHeaderPos"=w466:T24, "refnum out"=w495:refnum<file>)  [unwired: 3 in]
            n199 = call "HH_Start.vi"("Device Index"=w482, "Acq. Time"=w464, "error in (no error)"=w501) -> ("error out"=w457:errorcluster)  [unwired: 11 in, 1 out]
            n200 = Unbundle By Name(w457) -> ("status"=w510:bool)
            n201 = Not(x=w510) -> (.not. x?=w509:bool)
            n202 = case shown="True" w509 {
              tunnel: [w567 w590] -> w507
              tunnel: w457 -> [w568 w578]
              tunnel: w490 -> [w569 w589]
              tunnel: [w569 w588] -> w508
              tunnel: w482 -> [w562 w577]
              tunnel: w504 -> [_ w585]
              tunnel: w467 -> [_ w584]
              tunnel: [w566 w583] -> w503
              tunnel: [w566 w582] -> w502
              tunnel: w495 -> [w565 w581]
              tunnel: [w565 w580] -> w494
              tunnel: [i64 0 ("Num Records Total") w579] -> w493
              tunnel: [dbl[] [] w574] -> w452
              tunnel: [0 w573] -> w451
              frame False {
                (unwired) 0.0
                w566 = FALSE ("Stop Measurement")
                n203 = call "HH_Stop.vi"("Device Index"=w562, "error in (no error)"=w568) -> ("error out"=w567:errorcluster)  [unwired: 12 in, 1 out]
              }
              frame True {
                # "Overflow Interv. Time (s)"
                # "No Error"
                n204 = Initialize Array(0, 5) -> (w572:i32[])
                n205 = while {
                  tunnel: w577 -> [w599]
                  tunnel: w585 -> [w623]
                  tunnel: w584 -> [w622]
                  shift-right: [w600] -> w587
                  shift-left: w578 -> [w624]
                  shift-right: [w621] -> w588
                  shift-left: w589 -> [w621]
                  shift-right: [FALSE ("Reset")] -> _
                  shift-left: TRUE ("Reset") -> [w617]
                  tunnel: [w614] -> w583
                  tunnel: [w606] -> w582
                  tunnel: w581 -> [w610]
                  tunnel: [w609] -> w580
                  tunnel: [w608] -> w579
                  tunnel: [w607] -> w573
                  shift-right: [w594] -> w575
                  shift-left: w572 -> [w593]
                  tunnel: [w591] -> w576
                  i -> [w592]
                  stop <- w620 stop-if-true
                  n206 = call "HH_FIFORead.vi"("Device Index"=w599, "Buffer In"=w623, "Count"=w622, "error in (no error)"=w624) -> ("OK"=w615:bool, "Buffer Out"=w611:u32[], "Data Count"=w612:i32, "FiFo Overrun"=w614:bool, "error out"=w613:errorcluster)  [unwired: 7 in]
                  n207 = Wait (ms)(milliseconds to wait=u32 10) -> ()  [unwired: 1 out]
                  n208 = local write "Buffer Overrun"(w614) -> ()
                  n209 = Unbundle(w613) -> ("status"=w619:bool)  [unwired: 2 out]
                  n210 = call "HT3_Write.vi"("error in"=w613, "Data Count"=w612, "Data in"=w611, "refnum in"=w610) -> ("error out"=w601:errorcluster, "refnum out"=w609:refnum<file>)  [unwired: 6 in]
                  n211 = call "HH_TraceAndHisto.vi"("Data In"=w611, "Reset"=w617, "Data Count"=w612) -> ("Histograms"=w603:i32[][], "Total Oveflow Count"=w607:u64, "Num Records Total"=w608:i64, "Traces"=w602:i32[][])  [unwired: 8 in, 1 out]
                  n212 = local read "Stop Measurement"() -> (w605:bool)
                  n213 = local read "Global Stop"() -> (w604:bool)
                  n214 = local write "Trace"(w602) -> ()
                  n215 = call "GetCountRates.vi"("error in (no error)"=w601, "DeviceIndex"=w599) -> ("error out"=w600:errorcluster, "CntRates"=w595:dbl[], "SyncRate"=w596:i32)  [unwired: 1 in]
                  n216 = local write "Histogram"(w603) -> ()
                  n217 = Compound Arithmetic op=OR(invert w615, w619, w604, w605) -> (w620:bool)
                  n218 = Insert Into Array(array=w595, index=0, new element=w596) -> (w597:dbl[])
                  n219 = Or(x=w605, y=w604) -> (x .or. y?=w606:bool)
                  n220 = Add(x=w593, y=w597) -> (x+y=w594:dbl[])
                  n221 = Increment(x=w592) -> (x+1=w591:i32)
                }
                n222 = Divide(x=w575, y=w576) -> (x/y=w574:dbl[])
                n223 = call "HH_Stop.vi"("Device Index"=w577, "error in (no error)"=w587) -> ("error out"=w590:errorcluster)  [unwired: 12 in, 1 out]
              }
            }
            n224 = And(x=w462, y=w404) -> (x .and. y?=w461:bool)
            n225 = call "AOTF-Trigger_1.vi"("Channel"=w443, "Pulse length"=w434, "Sync trigger ratio"=5, "error in (no error)"=w455, "Triggered"=FALSE) -> ("error out"=w456:errorcluster)  [unwired: 2 in]
            n226 = call "PI Goto GPIB.vi"("System no."=w418, "x-position"=w421, "y-position"=w419, "z-position"=w420, "error in"=w423) -> ("error out"=w422:errorcluster)  [unwired: 14 in]
          }
          frame "Save Color Image" {
            n227 = local read "Active pt3"() -> (w633:path)
            n228 = call "MTS_GetFileFromWS.vi"(".pt3 File Name"=w633) -> ("File Header"=w632:T26)  [unwired: 9 in, 1 out]
            n229 = Unbundle By Name(w632) -> ("Measurement Type"=w631:T27, "Pixels"=w628:i32[])
            n230 = control-ref of="WS File Tree"() -> (w634:refnum<vi>)
            n231 = Equal?(x=T16."Image File" ("Measurement Type"), y=w631) -> (x = y?=w629:bool)
            n232 = case shown="True" w629 {
              tunnel: w638 -> [w639 w662]
              tunnel: w633 -> [_ w661]
              tunnel: w633 -> [_ _]
              tunnel: [w639 w641] -> w625
              tunnel: w634 -> [_ _]
              tunnel: w628 -> [_ w646]
              frame False {
              }
              frame True {
                # "Image Intensity Array"
                # "Image Intensity Array"
                n233 = call "HT3_Open.vi"("error in"=w662, "File Path"=w661) -> ("error out"=w654:errorcluster, "Header"=w658:T28, "refnum out"=w660:refnum<file>)  [unwired: 3 in, 4 out]
                n234 = Unbundle By Name(w658) -> ()  [unwired: 15 out]
                n235 = Index Array(array=w646, index #2=1 ("index")) -> (element #1=w643:i32, element #2=w644:i32)  [unwired: 1 in]
                n236 = Initialize Array(0 ("element"), w643, w644) -> (w656:i32[][])
                n237 = Initialize Array(0 ("element"), 4 ("dimension size"), w643, w644) -> (w649:i32[][][])
                n238 = while {
                  tunnel: w660 -> [w687]
                  shift-right: [FALSE ("Start From Top")] -> _
                  shift-left: TRUE ("Start From Top") -> [w681]
                  shift-right: [w680] -> w653
                  shift-left: w654 -> [w678]
                  tunnel: [w679] -> w652
                  tunnel: w656 -> [w677]
                  tunnel: [w676] -> w655
                  tunnel: [w677] -> _
                  stop <- w684 stop-if-true
                  n239 = call "HT3_Read.vi"("Start From Top"=w681, "error in"=w678, "Data count"=10000, "refnum in"=w687) -> ("error out"=w680:errorcluster, "Data out"=w683:u32[], "refnum out"=w679:refnum<file>, "EOF?"=w684:bool)  [unwired: 4 in]
                  n240 = Array Size(array=w683) -> (size(s)=w682:i32)
                  n241 = call "HH_FileToImage_1.vi"("Data In"=w683, "Reset"=w681, "Data Count"=w682) -> ("Histograms"=w676:i32[][])  [unwired: 7 in, 5 out]
                }
                n242 = call "MTS_SelectTCSPCBinning.vi"("Histograms in"=w655) -> ("TCSPC Binning"=w648:i32[][])  [unwired: 1 in, 9 out]
                n243 = while {
                  tunnel: w652 -> [w675]
                  shift-right: [FALSE ("Start From Top")] -> _
                  shift-left: TRUE ("Start From Top") -> [w669]
                  shift-right: [w668] -> w640
                  shift-left: w653 -> [w664]
                  tunnel: [w667] -> w642
                  tunnel: w649 -> [w666]
                  tunnel: [w665] -> _
                  tunnel: w648 -> [w663]
                  stop <- w672 stop-if-true
                  n244 = call "HT3_Read.vi"("Start From Top"=w669, "error in"=w664, "Data count"=10000, "refnum in"=w675) -> ("error out"=w668:errorcluster, "Data out"=w671:u32[], "refnum out"=w667:refnum<file>, "EOF?"=w672:bool)  [unwired: 4 out]
                  n245 = Array Size(array=w671) -> (size(s)=w670:i32)
                  n246 = call "HH_ToColorImage.vi"("Data In"=w671, "Reset"=w669, "Image Array In"=w666, "Data Count"=w670, "TCSPC Binning"=w663) -> ("Image Array Out"=w665:i32[][][])  [unwired: 2 in, 8 out]
                }
                n247 = Close File(refnum=w642, error in=w640) -> (error out=w641:errorcluster)  [unwired: 1 out]
              }
            }
          }
          frame "Find Single Mol." {
            n248 = local read "Active pt3"() -> (w706:path)
            n249 = call "MTS_GetFileFromWS.vi"(".pt3 File Name"=w706) -> ("File Header"=w705:T26)  [unwired: 9 in, 1 out]
            n250 = Unbundle By Name(w705) -> ("Measurement Type"=w704:T27, "Pixels"=w701:i32[], "Upper Left"=w700:T29, "Scan Axis"=w699:enum32{"x-y", "x-z", "y-z"})
            n251 = local read "Picture size Y"() -> (w691:dbl)
            n252 = local read "Picture size X"() -> (w692:dbl)
            n253 = Equal?(x=T16."Image File" ("Measurement Type"), y=w704) -> (x = y?=w702:bool)
            n254 = call "MTS_ScannerXYZToImageXY.vi"("Axis"=w699, "Scanner XYZ"=w700) -> ("Image Y"=w697:dbl, "Image X"=w698:dbl)
            n255 = Build Array(w692, w691) -> (w690:dbl[])
            n256 = case shown="True" w702 {
              tunnel: w696 -> [w707 w715]
              tunnel: w706 -> [_ _]
              tunnel: w706 -> [_ _]
              tunnel: [w707 w718] -> w693
              tunnel: w701 -> [_ w742]
              tunnel: w690 -> [_ w717]
              tunnel: w698 -> [_ w733]
              tunnel: w697 -> [_ w734]
              frame False {
              }
              frame True {
                w741 = 1 ("index")
                # "Gauss Width"
                # "Pixel Size [um]"
                n257 = Index Array(array=w717, index #2=w741) -> (element #1=w740:dbl, element #2=w736:dbl)  [unwired: 1 in]
                n258 = Index Array(array=w742, index #2=w741) -> (element #1=w739:i32, element #2=w737:i32)  [unwired: 1 in]
                n259 = Divide(x=w740, y=w739) -> (x/y=w730:dbl)
                n260 = Divide(x=w736, y=w737) -> (x/y=w735:dbl)
                n261 = local read "Image"() -> (w716:i32[][])
                n262 = Reciprocal(x=w730) -> (1/x=w729:dbl)
                n263 = Multiply(x=w729, y="psf width [um]") -> (x*y=w713:dbl)
                n264 = To Double Precision Float(number=w716) -> (double precision float=w712:dbl[][])
                n265 = script code="addpath(p);\nmask=GenGauss2D(gw);\n[err,bim,cim,sim,yc,xc,bc,cc,sc,len,imm]=FindPatternCP(image,mask,[],[],[],1.5);\nxc=xc-1;\nyc=yc-1;"("??"=w715, "gw"=w713, "image"=w712, "p"="C:\\Users\\Core-FCS\\Desktop\\Documents\\AbelFCS\\MatlabLibAbelFCS" ("String")) -> ("??"=w714:errorcluster, "xc"=w711:dbl[], "yc"=w710:dbl[])
                n266 = Multiply(x=w730, y=w711) -> (x*y=w732:dbl[])
                n267 = Multiply(x=w710, y=w735) -> (x*y=w731:dbl[])
                n268 = Add(x=w733, y=w732) -> (x+y=w722:dbl[])
                n269 = Add(x=w731, y=w734) -> (x+y=w721:dbl[])
                n270 = global read "patternImg.vi" "New Image"() -> (w708:T2)
                n271 = call "MTS_IntensityArrayToImage.vi"(0:"Image"=w708, 1:"Image"=w716, "error in (no error)"=w714, "Log Scale"=TRUE) -> ("Image Out"=w726:T2, "error out"=w727:errorcluster)  [unwired: 10 in]
                n272 = Build Array(w722, w721, w711, w710) -> (→"Pattern":dbl[][])
                n273 = for {
                  shift-right: [w749] -> w725
                  shift-left: w726 -> [w750]
                  tunnel: w711 -> [w748] mode=indexing
                  tunnel: w710 -> [w747] mode=indexing
                  shift-right: [w751] -> w719
                  shift-left: w727 -> [w752]
                  tunnel: u32 16738560 -> [w746]
                  tunnel: 3.0 ("x") -> [w745]
                  n274 = call "MTS_DrawCrossIMAQIamge.vi"("Image"=w750, "Size"=w745, "Color"=w746, "X"=w748, "Y"=w747, "error in (no error)"=w752) -> ("Image Out"=w749:T2, "error out"=w751:errorcluster)  [unwired: 8 in]
                }
                "AM image" <- w725
                n275 = flat-sequence {
                  tunnel: w719 -> [w744]
                  tunnel: [w744] -> w718
                  frame #0 {
                    n276 = local write item#-1(T19."AutoMesaurement" ("Tab Control")) -> ()
                  }
                }
              }
            }
          }
          frame "Auto Measurement Control" {
            # "Init"
            n277 = local read "NxtAutMesPoint"() -> (w762:i32)
            n278 = local read "Pattern"() -> (w767:dbl[][])
            n279 = Less Than 0?(x=w762) -> (x < 0?=w770:bool)
            n280 = Index Array(array=w767, index (row)=0) -> (element=w771:dbl[])  [unwired: 1 in]
            n281 = case shown="True" w770 {
              tunnel: w771 -> [_ w802]
              tunnel: w758 -> [w793 w797]
              tunnel: [w793 w796] -> w768
              tunnel: [w792 w794] -> w761
              frame False {
                n282 = local read "Auto Measure Points"() -> (w792:i32)
              }
              frame True {
                n283 = Array Size(array=w802) -> (size(s)=w794:i32)
                "Auto Measure Points" <- w794
                n284 = Number To Decimal String(number=w794) -> (decimal integer string=w799:string)  [unwired: 1 in]
                n285 = Concatenate Strings("Point 1 / " ("Caption.Text"), w799) -> (w798:string)
                n286 = property on="Auto Meas Progress" class="Slide (strict)"(error in=w797, "Scale.Minimum"=0.0 ("Scale.Range:Minimum"), "Scale.Maximum"=w794, "Value"=1 ("Auto Meas Progress"), "Caption.Text"=w798) -> (error out=w796:errorcluster)  [unwired: 1 in, 1 out]
              }
            }
            n287 = Increment(x=w762) -> (x+1=w760:i32)
            "NxtAutMesPoint" <- w760
            n288 = Increment(x=w760) -> (x+1=w759:i32)
            n289 = Index Array(array=w767, index (row) #1=2 ("index (row)"), index (col) #1=w760, index (row) #2=3 ("index (row)"), index (col) #2=w760) -> (element #1=w764:dbl, element #2=w763:dbl)
            n290 = Greater Or Equal?(x=w760, y=w761) -> (x >= y?=w769:bool)
            n291 = case shown="False" w769 {
              tunnel: w768 -> [w783 w791]
              tunnel: [w789 w791] -> w756
              tunnel: [T18."Auto Point" ("Do Measurement") T18."No Measurement" ("Do Measurement")] -> w755
              tunnel: w759 -> [w784 _]
              tunnel: w764 -> [w781 _]
              tunnel: w763 -> [w780 _]
              tunnel: w761 -> [w774 _]
              frame False {
                # "Prpare For Next Point"
                n292 = Number To Decimal String(number=w784) -> (decimal integer string=w786:string)  [unwired: 1 in]
                n293 = Number To Decimal String(number=w774) -> (decimal integer string=w775:string)  [unwired: 1 in]
                n294 = global read "patternImg.vi" "New Image"() -> (w773:T2)
                n295 = Concatenate Strings("Point " ("Caption.Text"), w786, " / " ("Caption.Text"), w775) -> (w785:string)
                n296 = call "MTS_DrawCrossIMAQIamge.vi"("Image"=w773, "Size"=3.0 ("x"), "Color"=u32 6618880, "X"=w781, "Y"=w780, "error in (no error)"=w783) -> ("Image Out"=w777:T2, "error out"=w782:errorcluster)  [unwired: 8 in]
                n297 = local write "AM image"(w777) -> ()
                n298 = property on="Auto Meas Progress" class="Slide (strict)"(error in=w782, "Value"=w784, "Caption.Text"=w785) -> (error out=w789:errorcluster)  [unwired: 1 in, 1 out]
              }
              frame True {
                # "No More Points"
              }
            }
          }
        }
      }
      frame Error {
      }
    }
    n299 = Unbundle(w114) -> ("status"=w113:bool)  [unwired: 2 out]
    n300 = flat-sequence {
      tunnel: w117 -> [w820]
      tunnel: [w820] -> w116
      tunnel: w112 -> [w817]
      tunnel: w110 -> [_]
      frame #0 {
        n301 = local write "Task"(w817) -> ()
        n302 = Equal?(x=w817, y=T12."No Measurement" ("Do Measurement")) -> (x = y?=w818:bool)
        n303 = Not(x=w818) -> (.not. x?=w819:bool)
        n304 = local write "Running"(w819) -> ()
      }
    }
    n305 = local read "Global Stop"() -> (w120:bool)
    n306 = Compound Arithmetic op=OR(w113, w118, w120) -> (w119:bool)
  }
  n307 = while {
    shift-right: [w840] -> w6
    shift-left: w16 -> [w842]
    stop <- w841 stop-if-true
    n308 = global read "GlobalLaserInterface.vi" "InterfaceLaserInitalised"() -> (w821:refnum<visa-resource-name>)
    n309 = control-ref of="WS File Tree"() -> (w826:refnum<vi>)
    n310 = event shown="[16] \"Resolution\", \"Picture size X\", \"Pixel time\", \"Picture size Y\", \"Axis\", \"CFD Settings.Laser  Profile\": Value Change" {
      selector: _ -> [_ _ _ _ _ _ _ _ _ _ _ _ _ _ _ _ _ _ _ _ _ _ _]
      dyn-events: _ -> [_ _ _ _ _ _ _ _ _ _ _ _ _ _ _ _ _ _ _ _ _ _ _]
      timeout: _ -> [_ _ _ _ _ _ _ _ _ _ _ _ _ _ _ _ _ _ _ _ _ _ _]
      tunnel: w842 -> [w843 w845 _ _ _ w918 _ _ _ _ w976 w1005 w1008 w1044 _ w1102 _ w1142 _ w1149 w1155 w1165 w1175]
      tunnel: [w843 w845 _ _ _ w918 _ _ _ _ w975 w1004 w1006 w1041 _ w1101 _ w1141 _ w1150 w1156 w1166 w1176] -> w840
      tunnel: w826 -> [_ _ _ _ _ _ _ _ _ _ _ _ w1010 w1045 _ _ _ _ _ _ _ _ _]
      tunnel: "Aquire Image" -> [_ _ _ _ _ _ _ _ _ _ _ _ _ _ _ _ _ _ _ _ _ _ _]
      tunnel: "Save Color Image" -> [_ _ _ _ _ _ _ _ _ _ _ _ _ _ _ _ _ _ _ _ _ _ _]
      tunnel: "Open MSW" -> [_ _ _ _ _ _ _ _ _ _ _ _ _ _ _ _ _ _ _ _ _ _ _]
      tunnel: "Find Mols" -> [_ _ _ _ _ _ _ _ _ _ _ _ _ _ _ _ _ _ _ _ _ _ _]
      tunnel: "Auto Meas" -> [_ _ _ _ _ _ _ _ _ _ _ _ _ _ _ _ _ _ _ _ _ _ _]
      tunnel: "Line Scan" -> [_ _ _ _ _ _ _ _ _ _ _ _ _ _ _ _ _ _ _ _ _ _ _]
      tunnel: "Grid Measurement" -> [_ _ _ _ _ _ _ _ _ _ _ _ _ _ _ _ _ _ _ _ _ _ _]
      tunnel: "New MSW" -> [_ _ _ _ _ _ _ _ _ _ _ _ _ _ _ _ _ _ _ _ _ _ _]
      tunnel: "Stop Program" -> [_ _ _ _ _ _ _ _ _ _ _ _ _ _ _ _ _ _ _ _ _ _ _]
      tunnel: "Point Measurement" -> [_ _ _ _ _ _ _ _ _ _ _ _ _ _ _ _ _ _ _ _ _ _ _]
      tunnel: "Move Stage" -> [_ _ _ _ _ _ _ _ _ _ _ _ _ _ _ _ _ _ _ _ _ _ _]
      tunnel: w821 -> [_ _ _ _ _ _ _ _ _ _ _ _ _ _ _ _ _ _ _ _ _ _ _]
      tunnel: "Get Position" -> [_ _ _ _ _ _ _ _ _ _ _ _ _ _ _ _ _ _ _ _ _ _ _]
      tunnel: [_ _ _ _ _ _ _ _ _ _ w971 w1002 _ _ _ _ _ _ _ _ _ _ _] -> w828
      tunnel: [_ _ _ _ _ _ _ _ _ _ w972 w1001 _ _ _ _ _ _ _ _ _ _ _] -> w825
      tunnel: [_ _ _ _ _ _ _ _ _ _ w973 w1000 _ _ _ _ _ _ _ _ _ _ _] -> w827
      tunnel: _ -> [_ _ _ _ _ _ _ _ _ _ _ _ _ _ _ _ _ _ w1148 _ _ _ _]
      tunnel: w826 -> [_ _ _ _ _ _ _ _ _ _ _ _ _ _ _ _ _ _ _ _ _ _ _]
      tunnel: "SCANNER EMERGENCY" -> [_ _ _ _ _ _ _ _ _ _ _ _ _ _ _ _ _ _ _ _ _ _ _]
      tunnel: "Auto Shutter Control" -> [_ _ _ _ _ _ _ _ _ _ _ _ _ _ _ _ _ _ _ _ _ _ _]
      event Timeout {
        n311 = event-data() -> ()  [unwired: 1 in, 2 out]
      }
      event "Stop Program": Mouse Up {
        n312 = event-data() -> ()  [unwired: 1 in, 7 out]
        n313 = local write "Global Stop"(TRUE ("Global Stop")) -> ()
      }
      event "Aquire Image": Mouse Up {
        n314 = event-data() -> ()  [unwired: 1 in, 7 out]
        n315 = local read "Workspace"() -> (w849:path)
        n316 = local read "Running"() -> (w852:bool)
        n317 = Not(x=w852) -> (.not. x?=w851:bool)
        n318 = Not Equal?(x=w849, y=path "") -> (x != y?=w847:bool)
        n319 = local read "Task"() -> (w846:T3)
        n320 = case shown="False" w847 {
          tunnel: w851 -> [_ w856]
          tunnel: T30."Aquire Image" ("Do Measurement") -> [_ w855]
          tunnel: w846 -> [_ w854]
          frame False {
            # "No Workspace Open"
            n321 = One Button Dialog(message="No Workspace Opened") -> ()  [unwired: 1 in, 1 out]
          }
          frame True {
            # "Aquire Image if not Running"
            n322 = case shown="False" w856 {
              tunnel: w855 -> [w859 w862]
              tunnel: w854 -> [w857 _]
              frame False {
                n323 = Equal?(x=w857, y=w859) -> (x = y?=w858:bool)
                n324 = case shown="True" w858 {
                  frame False {
                  }
                  frame True {
                    n325 = local write "Stop Measurement"(TRUE ("Stop Measurement")) -> ()
                  }
                }
              }
              frame True {
                n326 = local write "Task"(w862) -> ()
                n327 = local write "Running"(TRUE ("Measurement Running")) -> ()
                n328 = property on="Aquire Image" class="Bool"("BoolText.Text"="Stop Aquire" ("Caption.Text"), "BoolText.TextColor"=u32 16711680 ("Boolean Text.Colors:FG Color")) -> ()  [unwired: 2 in, 2 out]
              }
            }
          }
        }
      }
      event "Line Scan": Mouse Up {
        n329 = event-data() -> ()  [unwired: 1 in, 7 out]
        n330 = local read "Workspace"() -> (w868:path)
        n331 = local read "Running"() -> (w871:bool)
        n332 = Not(x=w871) -> (.not. x?=w870:bool)
        n333 = Not Equal?(x=w868, y=path "") -> (x != y?=w866:bool)
        n334 = local read "Task"() -> (w869:T3)
        n335 = case shown="False" w866 {
          tunnel: w870 -> [_ w875]
          tunnel: T31."Aquire Line Scan" ("Do Measurement") -> [_ w874]
          tunnel: w869 -> [_ w873]
          frame False {
            # "No Workspace Open"
            n336 = One Button Dialog(message="No Workspace Opened") -> ()  [unwired: 1 in, 1 out]
          }
          frame True {
            # "Aquire Image if not Running"
            n337 = case shown="False" w875 {
              tunnel: w874 -> [w877 w881]
              tunnel: w873 -> [w878 _]
              frame False {
                n338 = Equal?(x=w878, y=w877) -> (x = y?=w876:bool)
                n339 = case shown="True" w876 {
                  frame False {
                  }
                  frame True {
                    n340 = local write "Stop Measurement"(TRUE ("Stop Measurement")) -> ()
                  }
                }
              }
              frame True {
                n341 = local write "Task"(w881) -> ()
                n342 = local write "Running"(TRUE ("Measurement Running")) -> ()
                n343 = property on="Line Scan" class="Bool"("BoolText.Text"="Stop Scan" ("Caption.Text"), "BoolText.TextColor"=u32 16711680 ("Boolean Text.Colors:FG Color")) -> ()  [unwired: 2 in, 2 out]
              }
            }
          }
        }
      }
      event "Grid Measurement": Mouse Up {
        n344 = event-data() -> ()  [unwired: 1 in, 7 out]
        n345 = local read "Workspace"() -> (w891:path)
        n346 = local read "X-Position"() -> (w885:dbl)
        n347 = local read "Y-Position"() -> (w886:dbl)
        n348 = local read "Z-Position"() -> (w887:dbl)
        n349 = local read "Running"() -> (w894:bool)
        n350 = Build Array(w885, w886, w887) -> (w884:dbl[])
        n351 = Not(x=w894) -> (.not. x?=w893:bool)
        n352 = Not Equal?(x=w891, y=path "") -> (x != y?=w889:bool)
        n353 = local read "Task"() -> (w892:T3)
        n354 = case shown="True" w889 {
          tunnel: w893 -> [_ w899]
          tunnel: T12."Grid Measurement" ("Do Measurement") -> [_ w898]
          tunnel: w892 -> [_ w897]
          tunnel: w884 -> [_ w896]
          frame False {
            # "No Workspace Open"
            n355 = One Button Dialog(message="No Workspace Opened") -> ()  [unwired: 1 in, 1 out]
          }
          frame True {
            # "Aquire Grid if not Running"
            n356 = case shown="True" w899 {
              tunnel: w898 -> [w901 w915]
              tunnel: w897 -> [w902 _]
              tunnel: w896 -> [_ w905]
              frame False {
                n357 = Equal?(x=w902, y=w901) -> (x = y?=w900:bool)
                n358 = case shown="True" w900 {
                  frame False {
                  }
                  frame True {
                    n359 = local write "Stop Measurement"(TRUE ("Stop Measurement")) -> ()
                  }
                }
              }
              frame True {
                n360 = local write "Task"(w915) -> ()
                n361 = local write "Running"(TRUE ("Measurement Running")) -> ()
                n362 = local read "X-Axis Points"() -> (w910:u16)
                n363 = local read "Y-Axis Points"() -> (w909:u16)
                n364 = local read "Z-Axis Points"() -> (w908:u16)
                n365 = local read "X-Axis Offset"() -> (w913:dbl)
                n366 = local read "Y-Axis Offset"() -> (w912:dbl)
                n367 = local read "Z-Axis Offset"() -> (w911:dbl)
                n368 = property on="Grid Measurement" class="Bool"("BoolText.Text"="Stop Scan" ("Caption.Text"), "BoolText.TextColor"=u32 16711680 ("Boolean Text.Colors:FG Color")) -> ()  [unwired: 2 in, 2 out]
                n369 = Build Array(w910, w909, w908) -> (w906:u16[])
                n370 = Build Array(w913, w912, w911) -> (w904:dbl[])
                n371 = call "MTS_GenGridScanList.vi"("Offsets"=w904, "Points"=w906, "Starting"=w905) -> ("Grid Points"=w907:dbl[][])  [unwired: 8 in]
              }
            }
          }
        }
      }
      event "X-Axis Points", "Z-Axis Points", "Y-Axis Points": Value Change {
        n372 = event-data() -> ()  [unwired: 1 in, 5 out]
      }
      event "Auto Meas": Mouse Up {
        n373 = event-data() -> ()  [unwired: 1 in, 7 out]
        n374 = local read "Workspace"() -> (w926:path)
        n375 = local read item#-1() -> (w923)
        n376 = local read "Running"() -> (w929:bool)
        n377 = Not Equal?(x=w926, y=path "") -> (x != y?=w921:bool)
        n378 = Not Equal?(x=w923, y=-1) -> (x != y?=w920:bool)
        n379 = And(x=w921, y=w920) -> (x .and. y?=w919:bool)
        n380 = Not(x=w929) -> (.not. x?=w928:bool)
        n381 = local read "Task"() -> (w927:T3)
        n382 = case shown="False" w919 {
          tunnel: w928 -> [_ w933]
          tunnel: T18."Auto Measurement Control" ("Do Measurement") -> [_ w932]
          tunnel: w927 -> [_ w931]
          frame False {
            # "No Workspace Open"
            n383 = One Button Dialog(message="No Workspace Opened or No Image Acquired") -> ()  [unwired: 1 in, 1 out]
          }
          frame True {
            # "Start Auto Measurement"
            n384 = case shown="False" w933 {
              tunnel: w932 -> [_ w936]
              tunnel: w931 -> [_ _]
              frame False {
                n385 = case shown="True" FALSE {
                  frame False {
                  }
                  frame True {
                    n386 = local write "Stop Measurement"(TRUE ("Stop Measurement")) -> ()
                  }
                }
              }
              frame True {
                n387 = local write "Task"(w936) -> ()
                n388 = local write "Running"(TRUE ("Measurement Running")) -> ()
              }
            }
          }
        }
      }
      event "Save Color Image": Mouse Up {
        n389 = event-data() -> ()  [unwired: 1 in, 7 out]
        n390 = local read "Active pt3"() -> (w940:path)
        n391 = Not Equal?(x=w940, y=path "") -> (x != y?=w938:bool)
        n392 = case shown="True" w938 {
          tunnel: T32."Save Color Image" ("Do Measurement") -> [_ w944]
          frame False {
            # "No Workspace Open"
            n393 = One Button Dialog(message="No pt3 File opened") -> ()  [unwired: 1 in, 1 out]
          }
          frame True {
            # "Aquire Image if not Running"
            n394 = local write "Task"(w944) -> ()
            n395 = local write "Running"(TRUE ("Measurement Running")) -> ()
          }
        }
      }
      event "Find Mols": Mouse Up {
        n396 = event-data() -> ()  [unwired: 1 in, 7 out]
        n397 = local read "Active pt3"() -> (w947:path)
        n398 = Not Equal?(x=w947, y=path "") -> (x != y?=w945:bool)
        n399 = case shown="True" w945 {
          tunnel: T32."Find Single Mol." ("Do Measurement") -> [_ w951]
          frame False {
            # "No Workspace Open"
            n400 = One Button Dialog(message="No pt3 File opened") -> ()  [unwired: 1 in, 1 out]
          }
          frame True {
            # "Aquire Image if not Running"
            n401 = local write "Task"(w951) -> ()
            n402 = local write "Running"(TRUE ("Measurement Running")) -> ()
          }
        }
      }
      event "Point Measurement": Mouse Up {
        n403 = event-data() -> ()  [unwired: 1 in, 7 out]
        n404 = local read "Workspace"() -> (w954:path)
        n405 = local read "Running"() -> (w958:bool)
        n406 = Not(x=w958) -> (.not. x?=w957:bool)
        n407 = Not Equal?(x=w954, y=path "") -> (x != y?=w952:bool)
        n408 = local read "Task"() -> (w955:T3)
        n409 = case shown="True" w952 {
          tunnel: w957 -> [_ w962]
          tunnel: T30."Point Measurement" ("Do Measurement") -> [_ w961]
          tunnel: w955 -> [_ w960]
          frame False {
            # "No Workspace Open"
            n410 = One Button Dialog(message="No Workspace Opened") -> ()  [unwired: 1 in, 1 out]
          }
          frame True {
            # "Aquire Image if not Running"
            n411 = case shown="False" w962 {
              tunnel: w961 -> [w964 w968]
              tunnel: w960 -> [w965 _]
              frame False {
                n412 = Equal?(x=w965, y=w964) -> (x = y?=w963:bool)
                n413 = case shown="False" w963 {
                  frame False {
                  }
                  frame True {
                    n414 = local write "Stop Measurement"(TRUE ("Stop Measurement")) -> ()
                  }
                }
              }
              frame True {
                n415 = local write "Task"(w968) -> ()
                n416 = local write "Running"(TRUE ("Measurement Running")) -> ()
                n417 = property on="Point Measurement" class="Bool"("BoolText.Text"="Stop Aquire" ("Caption.Text"), "BoolText.TextColor"=u32 16711680 ("Boolean Text.Colors:FG Color")) -> ()  [unwired: 2 in, 2 out]
              }
            }
          }
        }
      }
      event "X-Position", "Y-Position", "Z-Position": Value Change; "Move Stage": Mouse Up {
        n418 = event-data() -> ()  [unwired: 1 in, 3 out]
        n419 = local read "Workspace"() -> (w979:path)
        n420 = local read "Running"() -> (w981:bool)
        n421 = local read "PI SystemNumber"() -> (w974:i32)
        n422 = Not(x=w981) -> (.not. x?=w980:bool)
        n423 = Not Equal?(x=w979, y=path "") -> (x != y?=w977:bool)
        n424 = case shown="True" w977 {
          tunnel: w980 -> [_ w989]
          tunnel: w976 -> [_ w988]
          tunnel: [_ w987] -> w975
          tunnel: w974 -> [_ w986]
          tunnel: [_ w985] -> w971
          tunnel: [_ w984] -> w972
          tunnel: [_ w983] -> w973
          frame False {
            # "No Workspace Open"
            n425 = One Button Dialog(message="No Workspace Opened") -> ()  [unwired: 1 in, 1 out]
          }
          frame True {
            # "Move Stage if not Running"
            n426 = case shown="True" w989 {
              tunnel: w988 -> [_ w996]
              tunnel: [_ w994] -> w987
              tunnel: w986 -> [_ w993]
              tunnel: [_ w992] -> w985
              tunnel: [_ w991] -> w984
              tunnel: [_ w990] -> w983
              frame False {
              }
              frame True {
                n427 = local read "X-Position"() -> (w999:dbl)
                n428 = local read "Y-Position"() -> (w998:dbl)
                n429 = local read "Z-Position"() -> (w997:dbl)
                n430 = call "PI Goto GPIB.vi"("System no."=w993, "x-position"=w999, "y-position"=w998, "z-position"=w997, "error in"=w996) -> ("error out"=w995:errorcluster)  [unwired: 14 in]
                n431 = call "PI Pos GPIB.vi"("System no."=w993, "error in"=w995) -> ("x-position"=w990:dbl, "y-position"=w991:dbl, "z-position"=w992:dbl, "error out"=w994:errorcluster)  [unwired: 14 in]
              }
            }
          }
        }
        n432 = property on="x-position" class="DigNum (strict)"("Value"=w973) -> ()  [unwired: 2 in, 2 out]
        n433 = property on="y-position" class="DigNum (strict)"("Value"=w972) -> ()  [unwired: 2 in, 2 out]
        n434 = property on="z-position" class="DigNum (strict)"("Value"=w971) -> ()  [unwired: 2 in, 2 out]
      }
      event "Get Position": Value Change {
        n435 = event-data() -> ()  [unwired: 1 in, 5 out]
        n436 = local read "PI SystemNumber"() -> (w1003:i32)
        n437 = call "PI Pos GPIB.vi"("System no."=w1003, "error in"=w1005) -> ("x-position"=w1000:dbl, "y-position"=w1001:dbl, "z-position"=w1002:dbl, "error out"=w1004:errorcluster)  [unwired: 14 in]
        n438 = property on="x-position" class="DigNum (strict)"("Value"=w1000) -> ()  [unwired: 2 in, 2 out]
        n439 = property on="y-position" class="DigNum (strict)"("Value"=w1001) -> ()  [unwired: 2 in, 2 out]
        n440 = property on="z-position" class="DigNum (strict)"("Value"=w1002) -> ()  [unwired: 2 in, 2 out]
      }
      event "New MSW": Mouse Up {
        # "Default Name"
        n441 = event-data() -> ()  [unwired: 1 in, 7 out]
        n442 = flat-sequence {
          tunnel: [w1026] -> w1009
          tunnel: w1008 -> [w1026]
          frame #0 {
            n443 = local write "Running"(TRUE ("MeasRunig")) -> ()
          }
        }
        n444 = Get Date/Time In Seconds() -> (seconds since 1Jan1904=w1023:timestamp)
        n445 = Format Date/Time String(time format string (%c)="%Y-%m-%d", seconds (now)=w1023) -> (date/time string=w1021:string)  [unwired: 1 out]
        n446 = Concatenate Strings(w1021, ".msw" ("string")) -> (w1019:string)
        n447 = call "File Dialog"("start path"=path "D:/", "prompt"="Create New Workspace", "button label"="Create", "default name"=w1019, "error in"=w1009, "pattern (all files)"="*.msw", "pattern label"="MT Scan Workspace") -> ("selected path"=w1013:path, "cancelled"=w1014:bool, "error out"=w1012:errorcluster)  [unwired: 5 in, 1 out]
        n448 = case shown="False" w1014 {
          tunnel: w1013 -> [w1032 _]
          tunnel: w1012 -> [w1038 w1040]
          tunnel: [w1030 w1039] -> w1007
          tunnel: w1010 -> [w1028 _]
          frame False {
            # "Create Empty Workspace"
            n449 = local write "Workspace"(w1032) -> ()
            n450 = call "MTS_CreateWriteMSW.vi"("Rewrite"=TRUE, "error in (no error)"=w1038, "Workspace Path"=w1032) -> ("error out"=w1031:errorcluster, "Created"=w1035:string, "Comment (dup)"=w1034:string, "Files in Workspace (dup)"=w1033:T34)  [unwired: 5 in]
            n451 = call "MTS_Workspace.vi"("Workspace"=w1032, "Operation"=T33."Set Workspace", "Created in"=w1035, "New Comment"=w1034, "Files in Workspace in"=w1033) -> ("Files in Workspace"=w1029:T35)  [unwired: 3 in, 3 out]
            n452 = call "MTS_BuildWSTree.vi"("error in"=w1031, "Files in Workspace"=w1029, "Tree Refnum"=w1028) -> ("error out"=w1030:errorcluster)  [unwired: 7 in, 1 out]
          }
          frame True {
            n453 = call <vilib>:"Clear Errors.vi"("error in (no error)"=w1040) -> ("error out"=w1039:errorcluster)  [unwired: 6 in]
          }
        }
        n454 = flat-sequence {
          tunnel: w1007 -> [w1024]
          tunnel: [w1024] -> w1006
          frame #0 {
            n455 = local write "Running"(FALSE ("MeasRunig")) -> ()
          }
        }
      }
      event "Open MSW": Mouse Up {
        n456 = event-data() -> ()  [unwired: 1 in, 7 out]
        n457 = flat-sequence {
          tunnel: w1044 -> [w1056]
          tunnel: [w1056] -> w1043
          frame #0 {
            n458 = local write "Running"(TRUE ("MeasRunig")) -> ()
          }
        }
        n459 = call "File Dialog2"("start path"=path "D:/", "prompt"="Create New Workspace", "button label"="Open", "error in"=w1043, "pattern (all files)"="*.msw", "pattern label"="MT Scan Workspace") -> ("selected path"=w1048:path, "cancelled"=w1049:bool, "error out"=w1047:errorcluster)  [unwired: 6 in, 1 out]
        n460 = case shown="False" w1049 {
          tunnel: w1048 -> [w1062 _]
          tunnel: w1047 -> [w1067 w1069]
          tunnel: [w1060 w1068] -> w1042
          tunnel: w1045 -> [w1058 _]
          frame False {
            # "Open Workspace"
            n461 = local write "Workspace"(w1062) -> ()
            n462 = call "MTS_ReadMSW.vi"("error in (no error)"=w1067, "Workspace Path"=w1062) -> ("error out"=w1061:errorcluster, "Created"=w1065:string, "Comment"=w1064:string, "Files in Workspace"=w1063:T36)  [unwired: 6 in]
            n463 = call "MTS_Workspace.vi"("Workspace"=w1062, "Operation"=T33."Set Workspace", "Created in"=w1065, "New Comment"=w1064, "Files in Workspace in"=w1063) -> ("Files in Workspace"=w1059:T35)  [unwired: 3 in, 3 out]
            n464 = call "MTS_BuildWSTree.vi"("error in"=w1061, "Files in Workspace"=w1059, "Tree Refnum"=w1058) -> ("error out"=w1060:errorcluster)  [unwired: 7 in, 1 out]
          }
          frame True {
            n465 = call <vilib>:"Clear Errors.vi"("error in (no error)"=w1069) -> ("error out"=w1068:errorcluster)  [unwired: 6 in]
          }
        }
        n466 = flat-sequence {
          tunnel: w1042 -> [w1054]
          tunnel: [w1054] -> w1041
          frame #0 {
            n467 = local write "Running"(FALSE ("MeasRunig")) -> ()
          }
        }
      }
      event "Image": Mouse Up {
        w1072 = 100.0 ("y")
        n468 = event-data() -> ("Coords"=w1084:T37, "PlatMods"=w1085:T38)  [unwired: 1 in, 5 out]
        n469 = invoke on="Image" class="IntGraph (strict)" method="Map Coords To XY"("Coords"=w1084) -> ("Map Coords To XY"=w1081:bool, "XY"=w1079:cluster{"X":dbl, "Y":dbl})  [unwired: 6 in, 5 out]
        n470 = Unbundle By Name(w1085) -> ("Ctrl"=w1082:bool)
        n471 = And(x=w1081, y=w1082) -> (x .and. y?=w1083:bool)
        n472 = Unbundle(w1079) -> ("X"=w1078:dbl, "Y"=w1075:dbl)
        n473 = Multiply(x=w1078, y=w1072) -> (x*y=w1077:dbl)
        n474 = Multiply(x=w1075, y=w1072) -> (x*y=w1074:dbl)
        n475 = Round To Nearest(number=w1077) -> (nearest integer value=w1076:dbl)
        n476 = Round To Nearest(number=w1074) -> (nearest integer value=w1073:dbl)
        n477 = Divide(x=w1076, y=w1072) -> (x/y=w1071:dbl)
        n478 = Divide(x=w1073, y=w1072) -> (x/y=w1070:dbl)
        n479 = local read "Axis"() -> (w1080:enum32{"x-y", "x-z", "y-x", "y-z", "z-x", "z-y"})
        n480 = case shown="True" w1083 {
          tunnel: w1080 -> [_ w1088]
          tunnel: w1071 -> [_ w1087]
          tunnel: w1070 -> [_ w1086]
          frame False {
          }
          frame True {
            n481 = case shown="\"x-y\", Default" w1088 {
              tunnel: w1087 -> [w1090 w1092 w1094]
              tunnel: w1086 -> [w1089 w1091 w1093]
              frame "x-y", Default {
                n482 = local write "X-Position"(w1090) -> ()
                n483 = local write "Y-Position"(w1089) -> ()
              }
              frame "x-z" {
                n484 = local write "X-Position"(w1092) -> ()
                n485 = local write "Z-Position"(w1091) -> ()
              }
              frame "y-z" {
                n486 = local write "Y-Position"(w1094) -> ()
                n487 = local write "Z-Position"(w1093) -> ()
              }
            }
          }
        }
      }
      event "WS File Tree": Value Change {
        n488 = event-data() -> ("NewVal"=w1103:string)  [unwired: 1 in, 4 out]
        n489 = control-ref of="Histogram"() -> (w1098:refnum<vi>)
        n490 = control-ref of="Trace"() -> (w1097:refnum<vi>)
        n491 = control-ref of="Image"() -> (w1096:refnum<vi>)
        n492 = control-ref of="Image"() -> (w1095:refnum<vi>)
        n493 = control-ref of="Workspace"() -> (w1100:refnum<vi>)
        n494 = control-ref of="Active pt3"() -> (w1099:refnum<vi>)
        n495 = call "CreateNewWSfile.vi"("reference 5"=w1095, "NewVal"=w1103, "Image"=w1096, "reference in"=w1099, "error in (no error)"=w1102, "reference 4"=w1097, "reference 3"=w1098, "Path in"=w1100) -> ("error out"=w1101:errorcluster)  [unwired: 3 in]
      }
      event "Resolution", "Picture size X", "Pixel time", "Picture size Y", "Axis", "CFD Settings.Laser  Profile": Value Change {
        n496 = event-data() -> ()  [unwired: 1 in, 5 out]
        n497 = local read "Pixel time"() -> (w1129:dbl)
        n498 = local read "Axis"() -> (w1126:enum32{"x-y", "x-z", "y-x", "y-z", "z-x", "z-y"})
        n499 = local read "Picture size Y"() -> (w1127:dbl)
        n500 = local read "Picture size X"() -> (w1128:dbl)
        n501 = local read "X-Position"() -> (w1123:dbl)
        n502 = local read "Y-Position"() -> (w1122:dbl)
        n503 = local read "Z-Position"() -> (w1121:dbl)
        n504 = local read item#-1() -> (w1110)
        n505 = local write "Axis"(w1126) -> ()
        n506 = local write "Pixel time"(w1129) -> ()
        n507 = local read "Resolution"() -> (w1120:dbl)
        n508 = call "PI_CheckScan.vi"("Picture size"=w1128, "Picture size 2"=w1127, "Axis"=w1126, "x-Position"=w1123, "y-Position"=w1122, "z-Position"=w1121) -> ("Picture size out"=w1124:dbl, "Picture size out 2"=w1125:dbl)  [unwired: 8 in, 4 out]
        n509 = String To Byte Array(string=w1110) -> (unsigned byte array=w1108:u8[])
        n510 = local write "Picture size X"(w1124) -> ()
        n511 = local write "Picture size Y"(w1125) -> ()
        n512 = Divide(x=w1124, y=w1120) -> (x/y=w1130:dbl)
        n513 = Divide(x=w1125, y=w1120) -> (x/y=w1131:dbl)
        n514 = Array Size(array=w1108) -> (size(s)=w1107:i32)
        n515 = Round Toward +Infinity(x=w1130) -> (ceil(x): smallest int >= x=→"Pixel X":dbl)
        n516 = Round Toward +Infinity(x=w1131) -> (ceil(x): smallest int >= x=→"Pixel Y":dbl)
        n517 = Initialize Array(4, w1107) -> (w1118:i32[])
        n518 = Initialize Array(1, w1107) -> (w1116:i32[])
        n519 = Subtract(x=w1108, y=48) -> (x-y=w1114:i32[])
        n520 = In Range and Coerce(upper limit=w1118, x=w1114, lower limit=w1116) -> (coerced(x)=w1111:i32[])  [unwired: 1 out]
        n521 = Add(x=w1111, y=48) -> (x+y=w1113:i32[])
        n522 = Byte Array To String(unsigned byte array=w1113) -> (string=w1109:string)
        n523 = while {
          shift-right: [w1136] -> w1106
          shift-left: w1109 -> [w1140]
          i -> [w1132]
          stop <- w1135 stop-if-true
          n524 = Increment(x=w1132) -> (x+1=w1133:i32)
          n525 = String Subset(string=w1140, offset (0)=w1132, length (rest)=1) -> (substring=w1138:string)
          n526 = Search and Replace String(replace all?=TRUE, input string=w1140, search string=w1138, offset=w1133) -> (result string=w1136:string)  [unwired: 4 in, 3 out]
          n527 = String Length(string=w1136) -> (length=w1134:i32)
          n528 = Less?(x=w1134, y=w1132) -> (x < y?=w1135:bool)
        }
        n529 = local write item#-1(w1106) -> ()
      }
      event "SCANNER EMERGENCY": Value Change {
        n530 = event-data() -> ()  [unwired: 1 in, 5 out]
        n531 = local read "PI SystemNumber"() -> (w1143:i32)
        n532 = call "PI Write GPIB.vi"("System no."=w1143, "String to send"="0RT", "error in"=w1142) -> ("error out"=w1145:errorcluster)  [unwired: 16 in]
        n533 = flat-sequence {
          tunnel: [w1146] -> w1141
          tunnel: w1145 -> [w1146]
          frame #0 {
            n534 = One Button Dialog(message="Emergency scanner stop appeared!!!\nCheck scanner settings before continue!!!") -> ()  [unwired: 2 out]
          }
        }
      }
      event "Measurement Time": Value Change {
        n535 = event-data() -> ()  [unwired: 1 in, 6 out]
        n536 = global write "GlobalSetGetConfigureCamera.vi" "Exposure"(w1148) -> ()
      }
      event "Stop Program": Value Change {
        n537 = event-data() -> ()  [unwired: 1 in, 6 out]
        n538 = flat-sequence {
          tunnel: w1149 -> [w1153]
          tunnel: [w1153] -> w1152
          frame #0 {
            n539 = local write "Global Stop"(TRUE ("Global Stop")) -> ()
          }
        }
        n540 = local read "PI SystemNumber"() -> (w1151:i32)
        n541 = call <userlib>:"Close connection if open.vi"("System no."=w1151, "error in"=w1152) -> ("error out"=w1150:errorcluster)  [unwired: 16 in, 1 out]
      }
      event "Excitation": Mouse Up {
        n542 = event-data() -> ()  [unwired: 1 in, 7 out]
        n543 = local read "Running"() -> (w1157:bool)
        n544 = Not(x=w1157) -> (.not. x?=w1158:bool)
        n545 = case shown="True" w1158 {
          tunnel: [_ w1159] -> w1156
          tunnel: w1155 -> [_ w1159]
          frame False {
          }
          frame True {
            n546 = local read "Detector 1"() -> (w1161:bool)
            n547 = local read "Detector 2"() -> (w1160:bool)
            n548 = local read "Excitation"() -> (w1163:bool)
            n549 = Not(x=w1163) -> (.not. x?=w1162:bool)
            n550 = call "PCAN_CompMessage.vi"("Detector2"=w1160, "Detector1"=w1161, "Excitation"=w1162) -> ("CAN_Message"=w1164:T39)
            n551 = call "CAN USB Write.vi"("CAN_Message"=w1164) -> ()  [unwired: 2 in, 1 out]
          }
        }
      }
      event "Detector 1": Mouse Up {
        n552 = event-data() -> ()  [unwired: 1 in, 7 out]
        n553 = local read "Running"() -> (w1167:bool)
        n554 = Not(x=w1167) -> (.not. x?=w1168:bool)
        n555 = case shown="True" w1168 {
          tunnel: [_ w1169] -> w1166
          tunnel: w1165 -> [_ w1169]
          frame False {
          }
          frame True {
            n556 = local read "Detector 1"() -> (w1172:bool)
            n557 = local read "Detector 2"() -> (w1173:bool)
            n558 = local read "Excitation"() -> (w1170:bool)
            n559 = Not(x=w1172) -> (.not. x?=w1171:bool)
            n560 = call "PCAN_CompMessage.vi"("Detector2"=w1173, "Detector1"=w1171, "Excitation"=w1170) -> ("CAN_Message"=w1174:T39)
            n561 = call "CAN USB Write.vi"("CAN_Message"=w1174) -> ()  [unwired: 2 in, 1 out]
          }
        }
      }
      event "Detector 2": Mouse Up {
        n562 = event-data() -> ()  [unwired: 1 in, 7 out]
        n563 = local read "Running"() -> (w1177:bool)
        n564 = Not(x=w1177) -> (.not. x?=w1178:bool)
        n565 = case shown="True" w1178 {
          tunnel: [_ w1179] -> w1176
          tunnel: w1175 -> [_ w1179]
          frame False {
          }
          frame True {
            n566 = local read "Detector 1"() -> (w1182:bool)
            n567 = local read "Detector 2"() -> (w1180:bool)
            n568 = local read "Excitation"() -> (w1183:bool)
            n569 = Not(x=w1180) -> (.not. x?=w1181:bool)
            n570 = call "PCAN_CompMessage.vi"("Detector2"=w1181, "Detector1"=w1182, "Excitation"=w1183) -> ("CAN_Message"=w1184:T39)
            n571 = call "CAN USB Write.vi"("CAN_Message"=w1184) -> ()  [unwired: 2 in, 1 out]
          }
        }
      }
    }
    "z-position" <- w828
    "y-position" <- w825
    "x-position" <- w827
    n572 = local read "Global Stop"() -> (w841:bool)
  }
  n573 = call "DT3120_CloseDevice.vi"("error in (no error)"=w9) -> ("error out"=w11:errorcluster)  [unwired: 1 in, 9 out]
  n574 = call "IMAQ Dispose"("Image"=w8, "error in (no error)"=w11) -> ("error out"=w10:errorcluster)  [unwired: 4 in]
  n575 = flat-sequence {
    tunnel: w10 -> [w1187]
    tunnel: [w1185] -> w7
    frame #0 {
      n576 = call "CAN USB Close.vi"() -> ("Error Number"=w1186:u32)  [unwired: 1 in]
      n577 = call <vilib>:"Error Cluster From Error Code.vi"("error in (no error)"=w1187, "error message (\"\")"="PCAN Close Error" ("error message (\"\")"), "error code (0)"=w1186) -> ("error out"=w1185:errorcluster)  [unwired: 6 in]
    }
  }
  n578 = Merge Errors(w7, w6) -> (w5:errorcluster)
  n579 = Divide(x=w24, y=w23) -> ()  [unwired: 1 out]
  n580 = flat-sequence {
    tunnel: w2 -> [w1190]
    tunnel: [w1190] -> w1
    frame #0 {
      n581 = local write "Global Stop"(TRUE ("Global Stop")) -> ()
    }
  }
  n582 = global read "patternImg.vi" "New Image"() -> (w15:T2)
  n583 = call "IMAQ Dispose"("Image"=w15, "error in (no error)"=w1) -> ("error out"=w3:errorcluster)  [unwired: 4 in]
  n584 = Merge Errors(w5, w3) -> (→"error out":errorcluster)
  n585 = Divide(x=32767.0 ("Maximum Voltage"), y=3276.8) -> ()  [unwired: 1 out]
